vi "DB UI - Master Data Layout.vi"() -> ()   [LabVIEW 2013]
uses:
  Controls/Output Set Cluster.ctl
  Controls/Combo Box.ctl
  <vilib>/Utility/miscctls.llb/LVRowAndColumnUnsignedTypeDef.ctl
  <vilib>/Utility/miscctls.llb/LVRowAndColumnTypeDef.ctl
  <vilib>/Utility/miscctls.llb/LVPointTypeDef.ctl
  Controls/DB - Master Data Layout Enum.ctl
  Controls/DB - [MasterData].[OutputSet] ColNames.ctl
  Controls/Global SRTRS.vi
  <vilib>/addons/database/Connection.llb/DB Tools Open Connec (String).vi
  <vilib>/addons/database/Connection.llb/Conn Execute.vi
  <vilib>/addons/database/Recordset.llb/Rec Destroy - Connection.vi
  <vilib>/addons/database/Recordset.llb/Rec Fetch Recordset Data (R).vi
  <vilib>/addons/database/_DB Variant To Data/Database Variant To Data.xnode
  <vilib>/addons/database/NI_Database_API.lvlib
  Controls/Message Code - Enum.ctl
panel:
  in  "Tab Control":enum32{"Debug"}(tab)
  out "MHandler":errorcluster
  in  "Stop Button":bool
  out "Statemachine":errorcluster
  in  "# of Columns":i32=8
  out "Primary Keys":string[](array[string])=["OrderNo"]
  out "Foreign Keys":string[](array[string])=["OrderNo"]
  out "Record Count":i32
  in  "Next Button":bool
  in  "Previous Button":bool
  in  "Current Record":i32
  out "1st Primary KEY":string
  in  "Last Button":bool
  in  "First Button":bool
  out "datetime string":string
  out "Output Set Changed":bool
  in  "Include Inactive":bool=TRUE
  out "Extra Event From \"Select Foreign Key\" (NA)":bool
  out "IDENTITY COLUMN":string
  out "Close":errorcluster
  out "New Record in UI not in DB (NA)":bool
  out "Property Node":errorcluster
  out "DB":errorcluster
  in  "SRTRS.MasterData.OutputSet":string="SRTRS.MasterData.OutputSet"
  in  "[PlantId]":string="4070"
  in  "SRTRS.MasterData.OutputLayout":string="SRTRS.MasterData.OutputLayout"
  in  "SRTRS.Config.OutputType":string="SRTRS.Config.OutputType"
  out "Col Hdrs[] DB Data Type":string[](array[string])
  in  "Search User ID":T1
  in  "# of Rows":u32=5
  out "Col Hdrs[] DB Precision":string[](array[string])
  out "All Mandatory Fields Filled":bool
  in  "------------------------------------        Layout Details EVENTS     ------------------------------------":string caption="------------------------------------        Setup Tab     ------------------------------------"
  in  "------------------------------------------        Unused EVENTS     ----------------------------------------":string caption="------------------------------------        Setup Tab     ------------------------------------"
  out "Connection Information":T2={"Connection "="SQL Server 32bit HPEnvy", "Username"="admin", "Password"="admin123"}
  out "[Column Name] Changed":string
  out "File":errorcluster
  out "Editing Layout Details in New Record":bool
  in  "------------------------------------        Header EVENTS     ------------------------------------   2":string caption="------------------------------------        Setup Tab     ------------------------------------"
  in  "------------------------------------        MCListBox EVENTS     ------------------------------------   3":string caption="------------------------------------        Setup Tab     ------------------------------------"
  out "Precision":i32
  out "SQL":string[](array[string])
  in  "SRTRS.MasterData.Layout":string="SRTRS.MasterData.Layout"
  out "New Layout Id":string[](array[string])
  out "Source path":path caption="selected path"
  out "Target path":path
  out "File Copy Error":errorcluster
  out "MCListBox":u32
  out "NewVal":i32
  out "Layout Details":u32
  in  "Add (Not Save) Enabled depends on \nFilled Mandatory Fields":bool=TRUE
  out "Empty ColHdrs[]":string[](array[string])
  in  "UPDATE ALL LayoutId":bool=TRUE
  in  "CellBG New Cells":u32(colorbox)=16777225
  in  "CellBG Unused Cells":u32(colorbox)=16777238
  in  "CellBG ColHdrs":u32(colorbox)=11776947
  in  "New Layout ID":bool
  in  "Output Set Header":T3 caption="Header"
  in  "Layout Browse":bool caption="Material Browse"
  in  "Item Number":i32=1 min=0 step=1
  in  "Layout Details Cluster":T4 caption="Layout Details"
  in  "Delete":bool caption="Setup Save"
  in  "Add":bool caption="Setup Save"
  in  "Save":bool caption="Setup Save"
  in  "New":bool caption="Setup Save"
  in  "MCListbox Layout":i32(listbox)=3 caption="MCListBox Layout"
  # "No."
  # "/"
  # "Record"
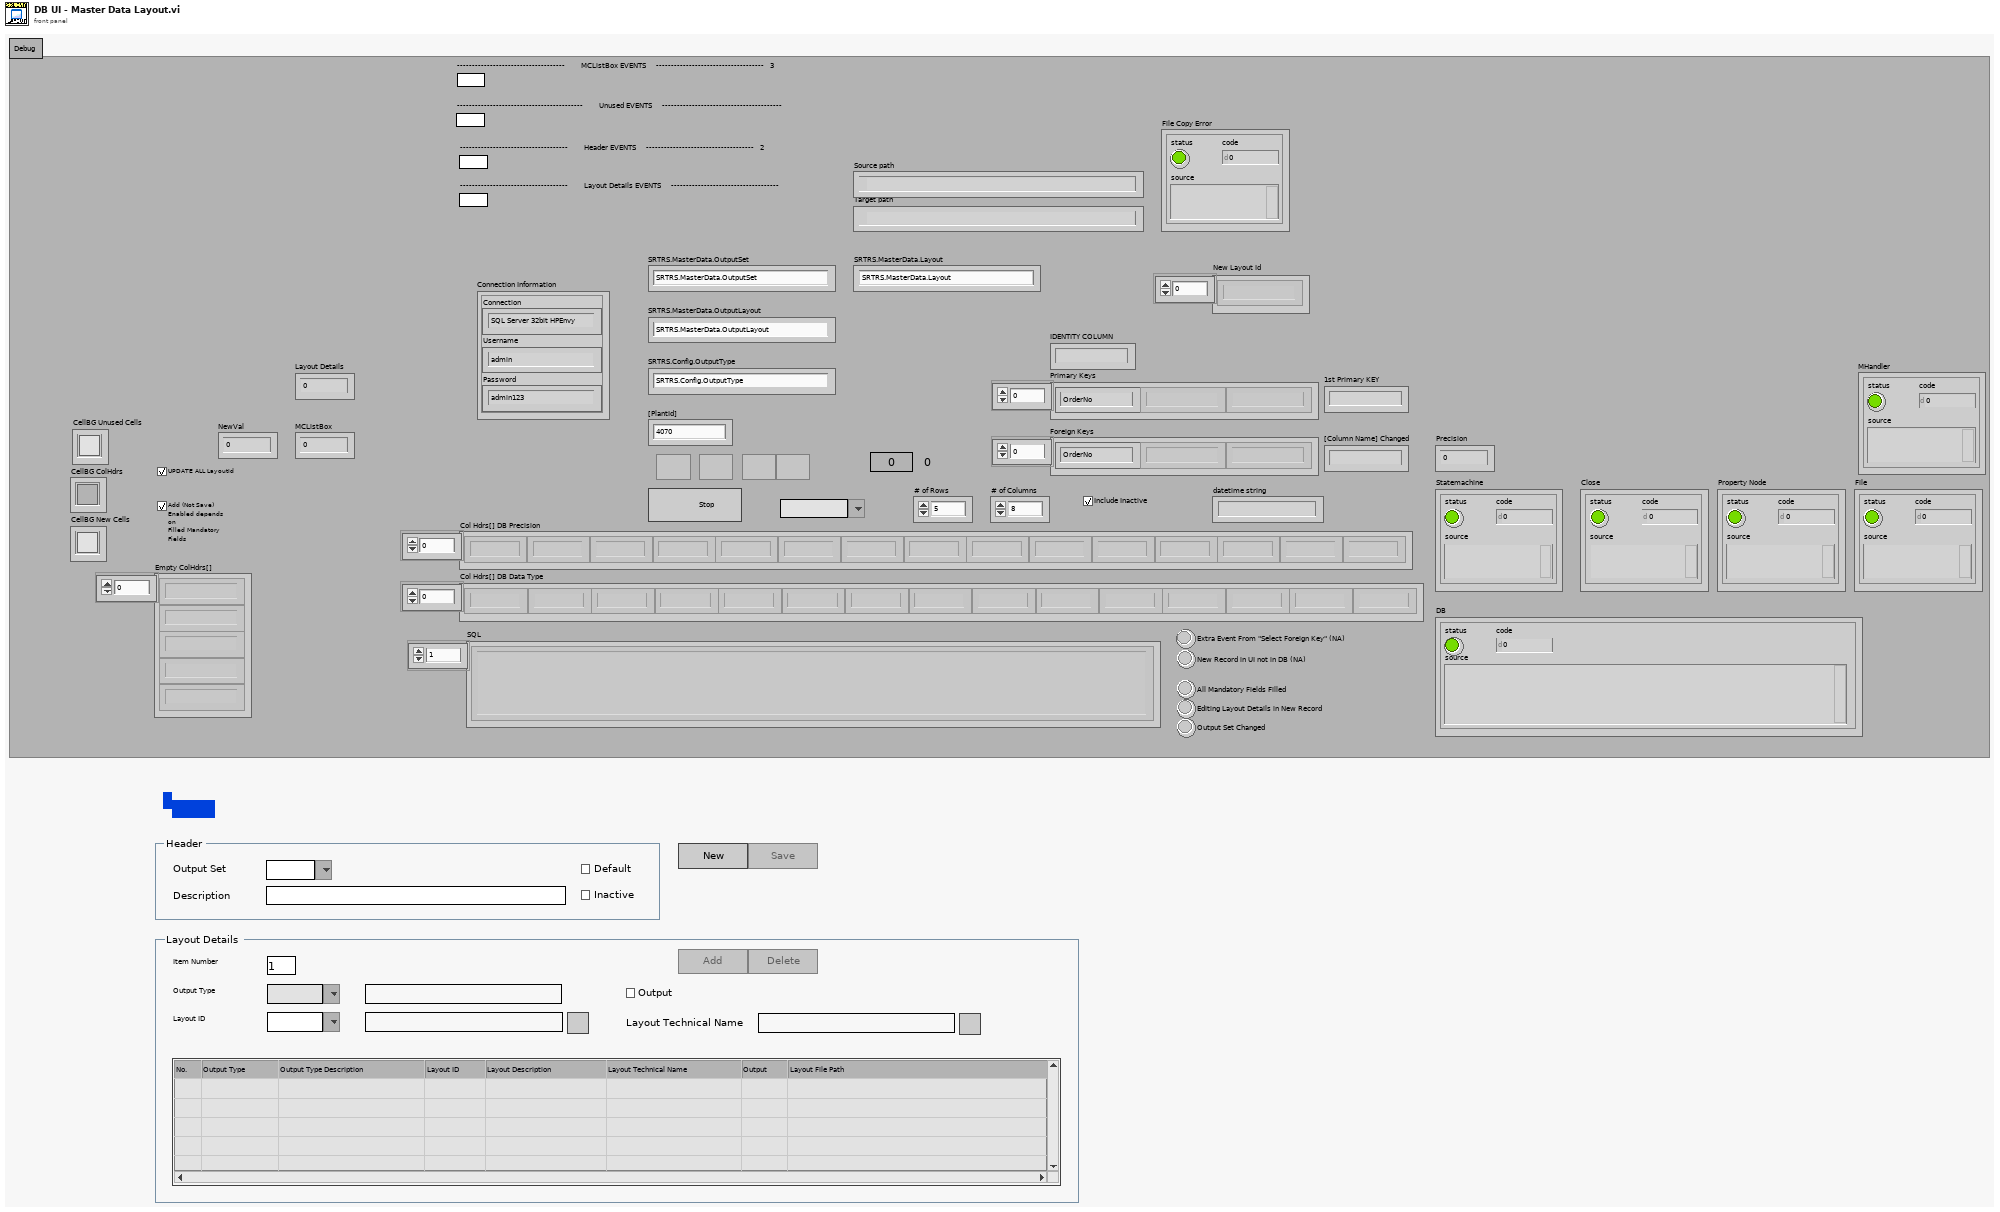
[diagram p1: front panel]
types:
  T1 = typedef "Combo Box.ctl" = string
  T2 = cluster{"Connection ":string, "Username":string, "Password":string}
  T3 = typedef "Output Set Cluster.ctl" = cluster{"Output Set":T1, "Description":string, "Default":bool, "Inactive":bool}
  T4 = cluster{"Output Type":T1, "Output":bool, "Inactive":bool, "Layout Description":string, "Layout ID":T1, "Layout Technical Name":string, "Output Type Description":string, "Layout File Path":string}
  T5 = enum8{"Enabled", "Disabled", "Disabled and Grayed Out"}
  T6 = typedef "LVPointTypeDef.ctl" = cluster{"Horizontal":i16, "Vertical":i16}
  T7 = typedef "LVRowAndColumnUnsignedTypeDef.ctl" = cluster{"Row":u32, "Column":u32}
  T8 = typedef "DB - Master Data Layout Enum.ctl" = enum16{"b.[ItemNo]", "a.[OutputSetId]", "a.[Description]", "a.[Default]", "a.[Inactive]", "b.[OutputTypeId]", "c.[ShortDescription]", "b.[Output]", "b.[Inactive]", "b.[LayoutId]", "b.[Description]", "b.[LayoutFileName]", "b.[LayoutFilePath]"}
  T9 = typedef "LVRowAndColumnTypeDef.ctl" = cluster{"Row":i32, "Column":i32}
  T10 = typedef "DB - Logon Info.ctl" = cluster{"PlantID":string, "SystemID":string, "UserID":string, "DomainID":string, "LanguageID":string, "StationID":string}
  T11 = typedef "Connection Information Cluster.ctl" = cluster{"Connection ":string, "Username":string, "Password":string}
  T12 = typedef "NI_Database_API.lvlib/Conn ObjectReference.ctl" = refnum<k1>
  T13 = typedef "Message Code - Enum.ctl" = enum16{"<APP><I 100>", "<APP><E 101>", "<APP><I 110>", "<APP><W 111>", "<APP><I 112>", "<APP><W 113>", "<APP><I 114>", "<APP><I 115>", "<APP><I 116>", "<APP><W 117>", "<APP><I 120>", "<APP><W 121>", "<APP><E 122>", "<APP><W 130>", "<APP><W 131>", "<APP><W 132>", "<APP><W 133>", "<APP><W 134>", "<DB><I 150>", "<DB><I 151>", "<DB><W 152>", "<APP><I 200>", "<APP><I 201>", "<APP><W 202>", "<APP><E 203>", "<DB><I 300>", "<DB><I 301>", "<DB><W 302>", "<DB><I 305>", "<DB><I 306>", "<DB><W 307>", "<DB><W 310>", "<cRIO><I 400>", "<cRIO><W 401>", "<cRIO><I 402>", "<cRIO><W 403>", "<ET><I 500>", "<ET><W 501>", "<ET><I 600>", "<ET><W 601>", "<ET><E 602>", "<ET><I 610>", "<ET><W 611>", "<ET><E 612>"}
  T14 = typedef "DB - [MasterData].[OutputSet] ColNames.ctl" = enum16{"[PlantId]", "[OutputSetId]", "[Description]", "[Default]", "[CreatedBy]", "[CreatedOn]", "[LastSavedBy]", "[LastSavedOn]", "[Inactive]"}
  T15 = typedef "DB - DB.Schema.Table.ctl" = cluster{"DB":string, "Schema":string, "Table":string}
  T16 = typedef "NI_Database_API.lvlib/Rec ObjectReference.ctl" = refnum<k1>
  T17 = cluster{"Output Set":T1, "Description":string, "Default":bool, "Inactive":bool}
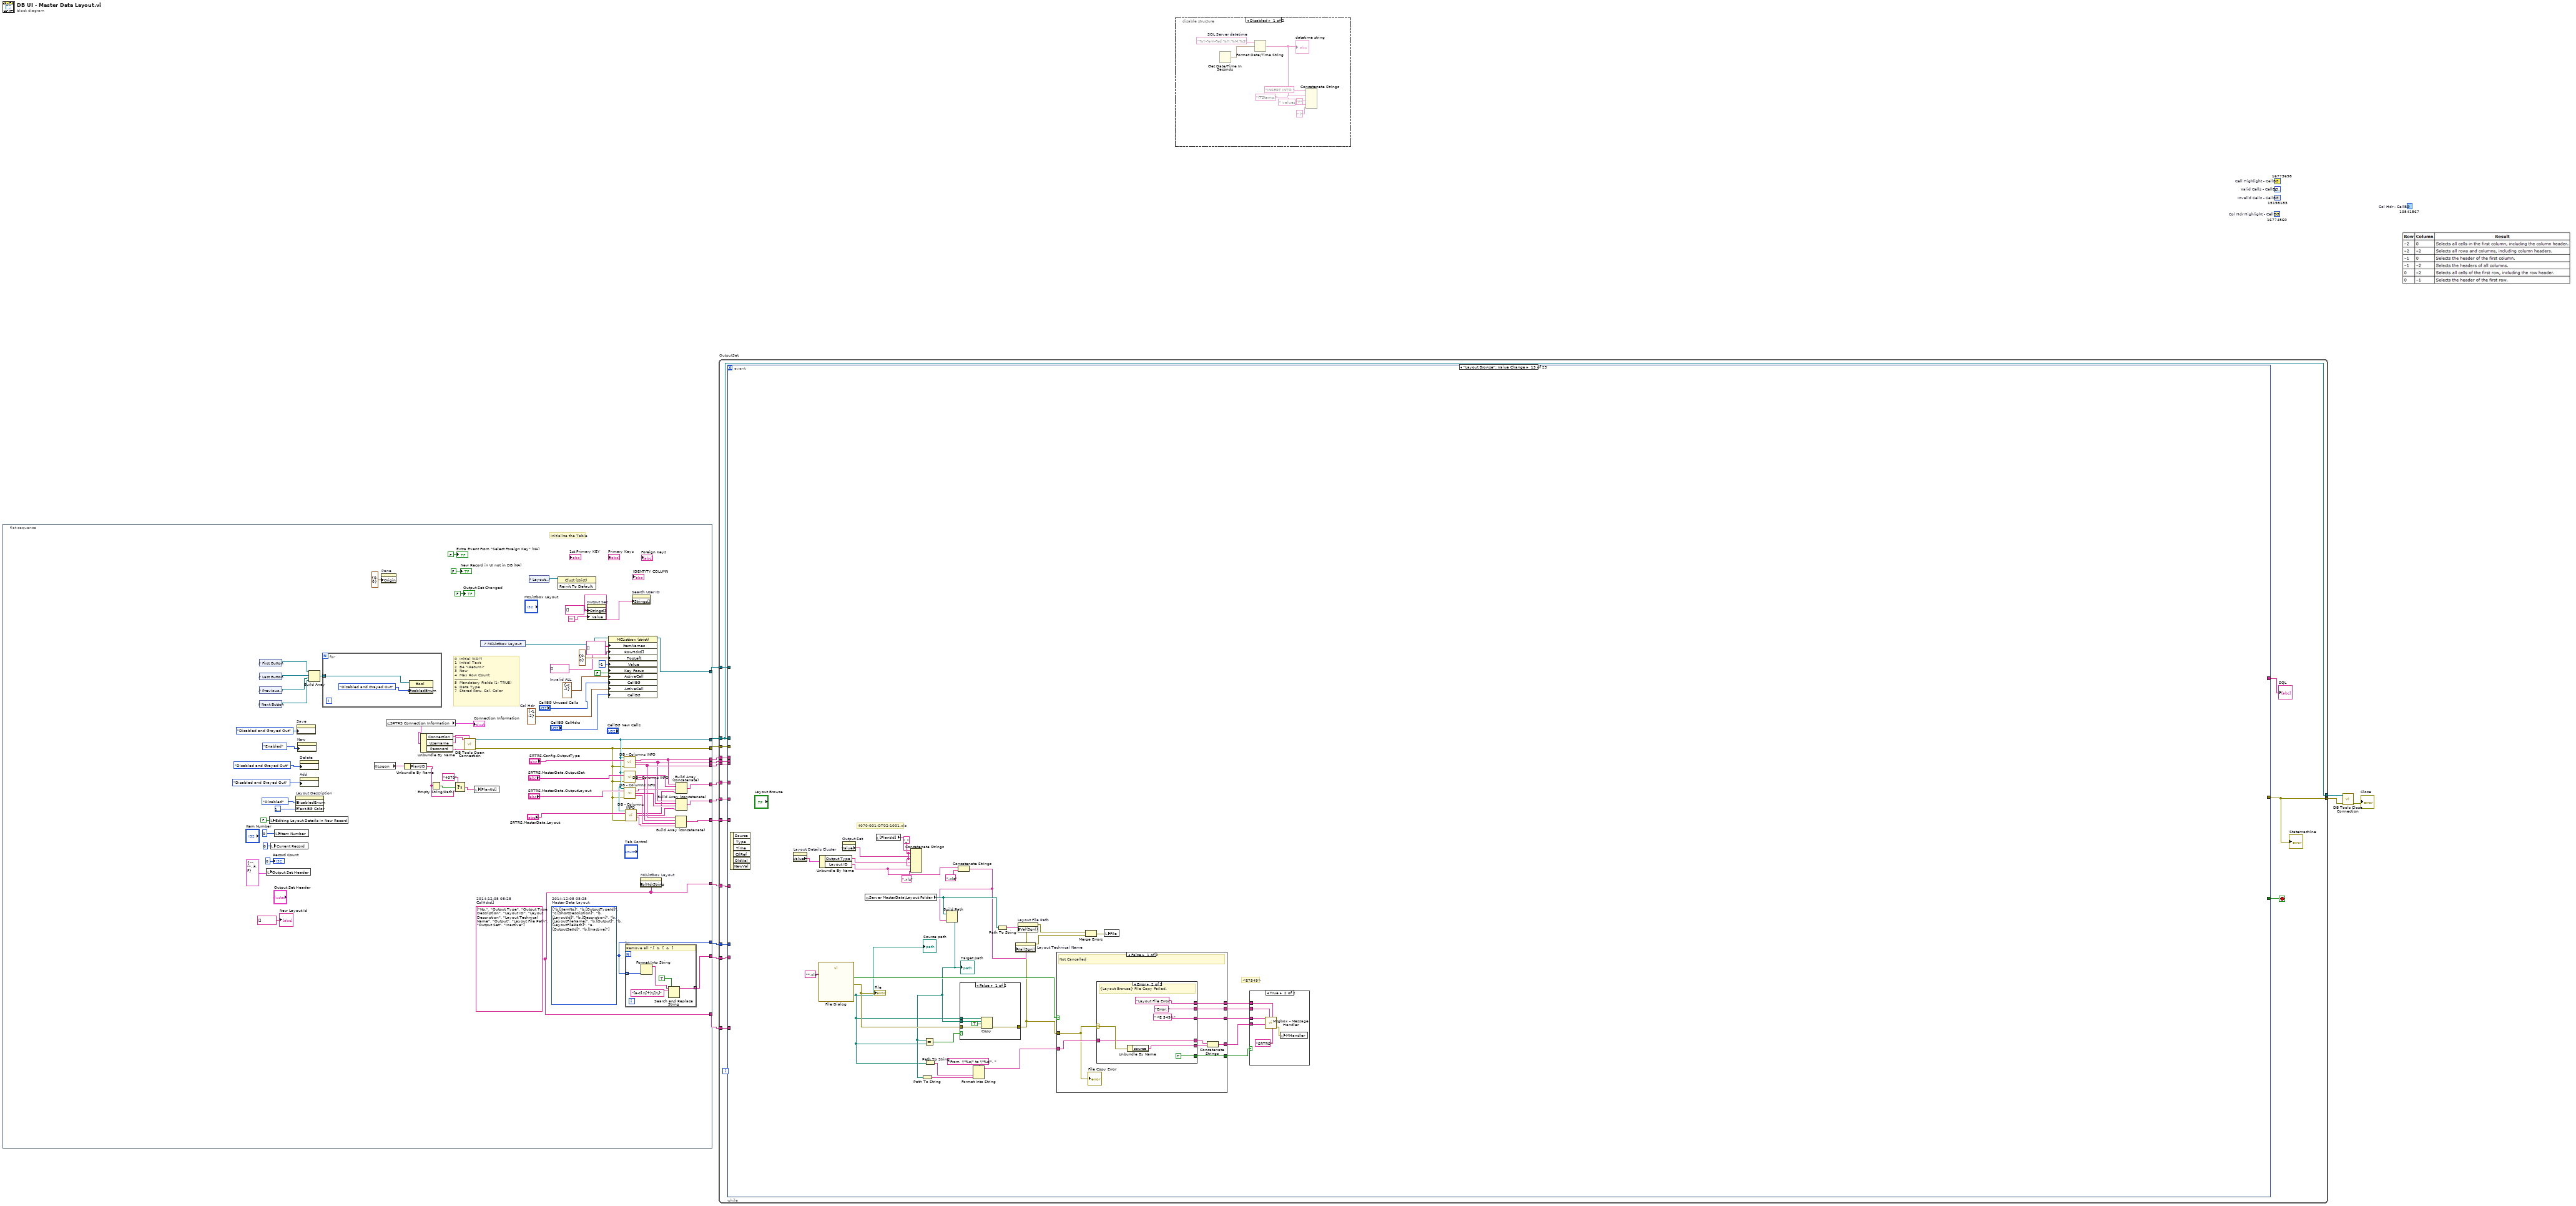
[diagram p0: block diagram]
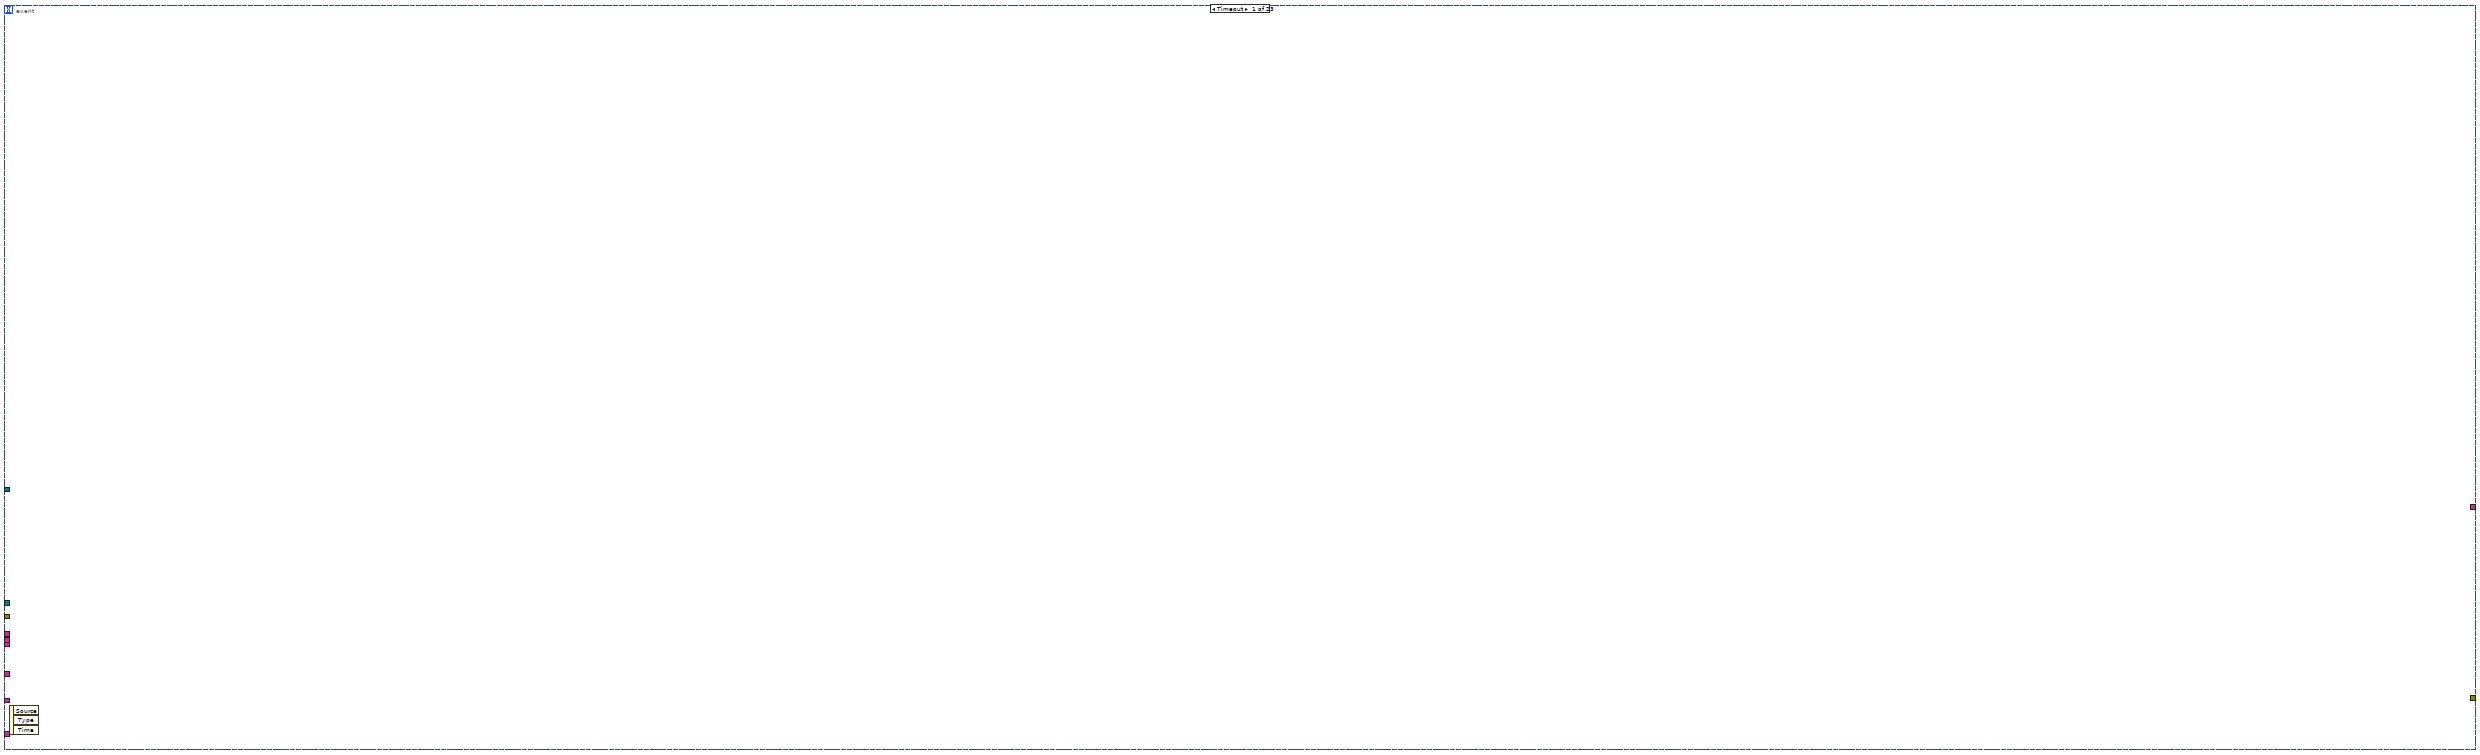
[diagram p3: hidden frame]
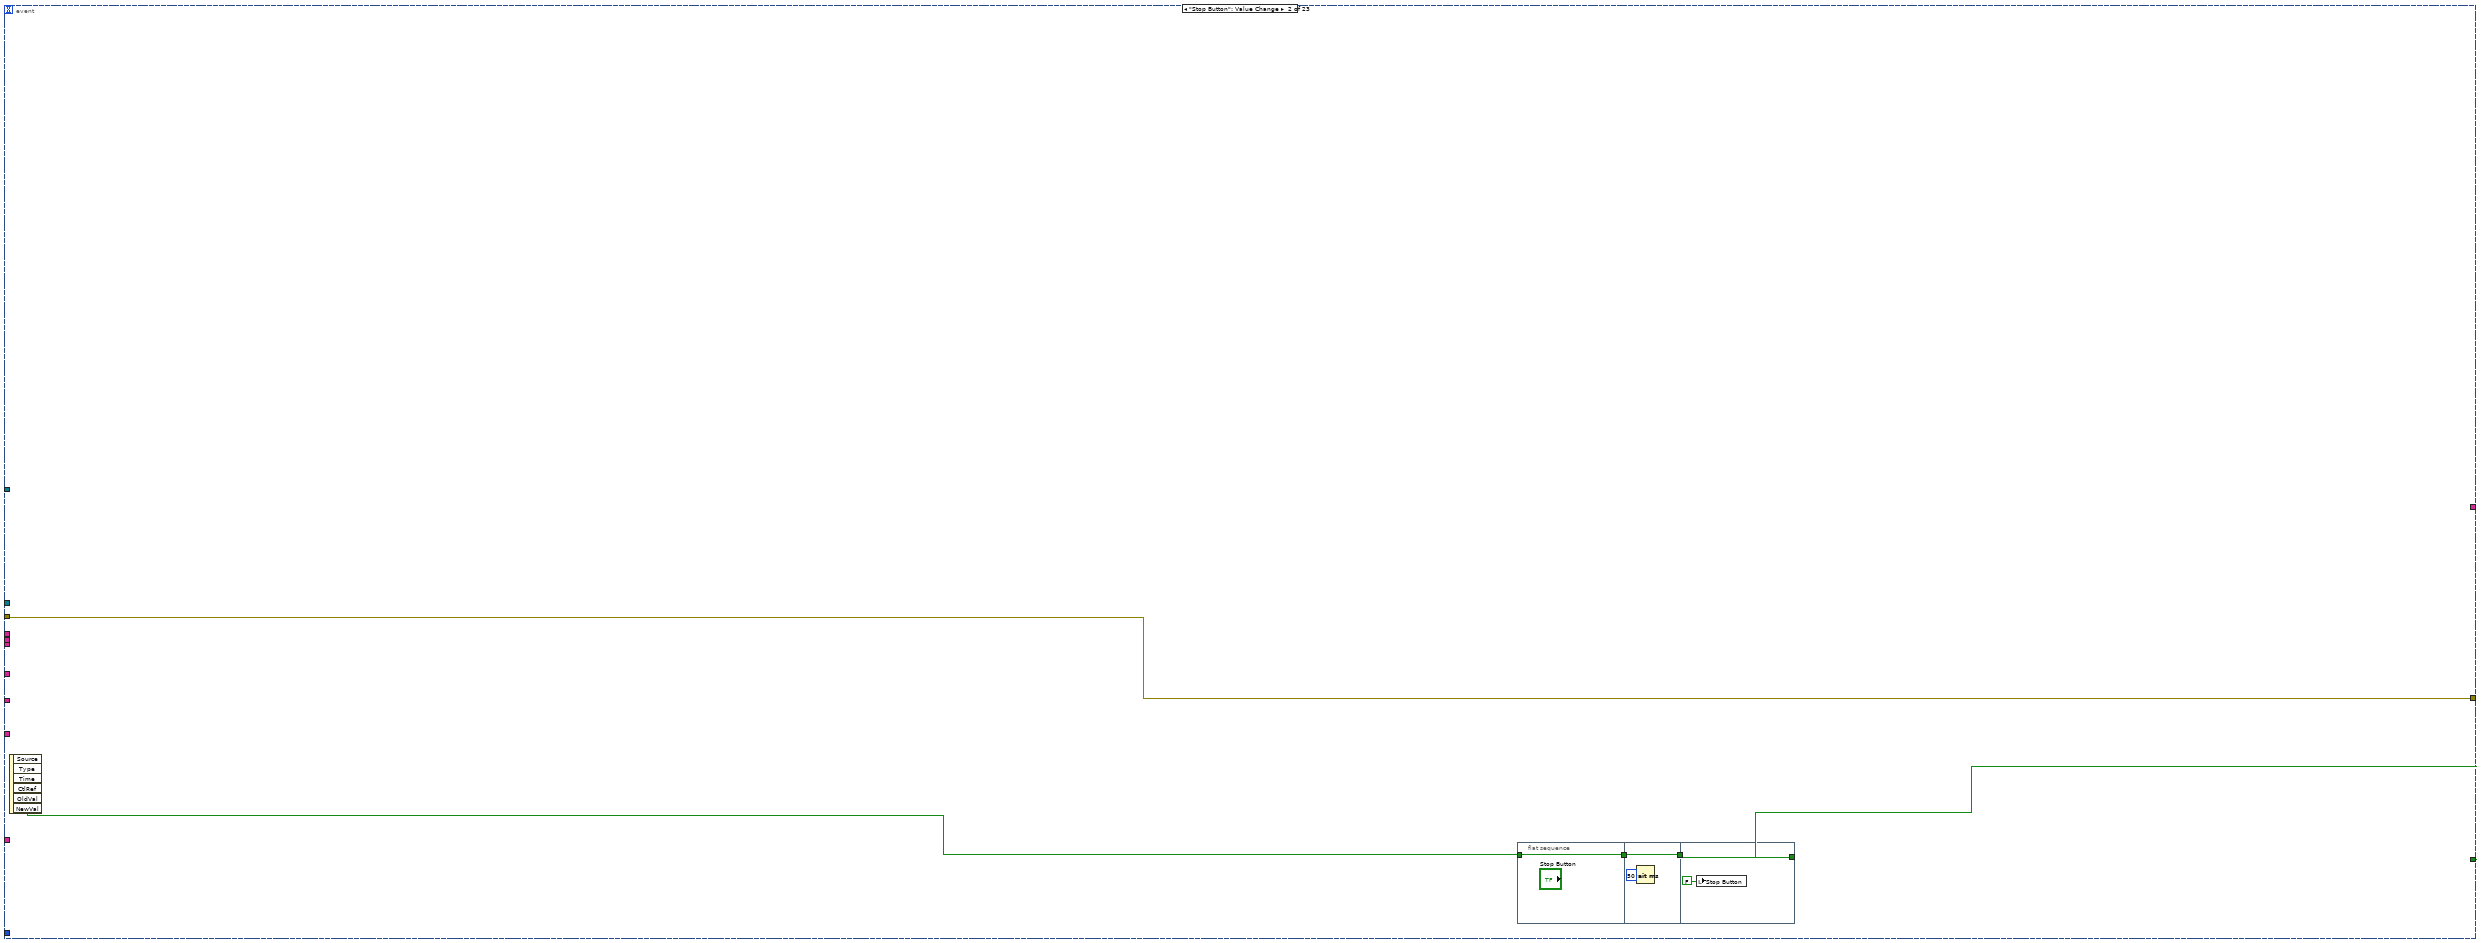
[diagram p4: hidden frame]
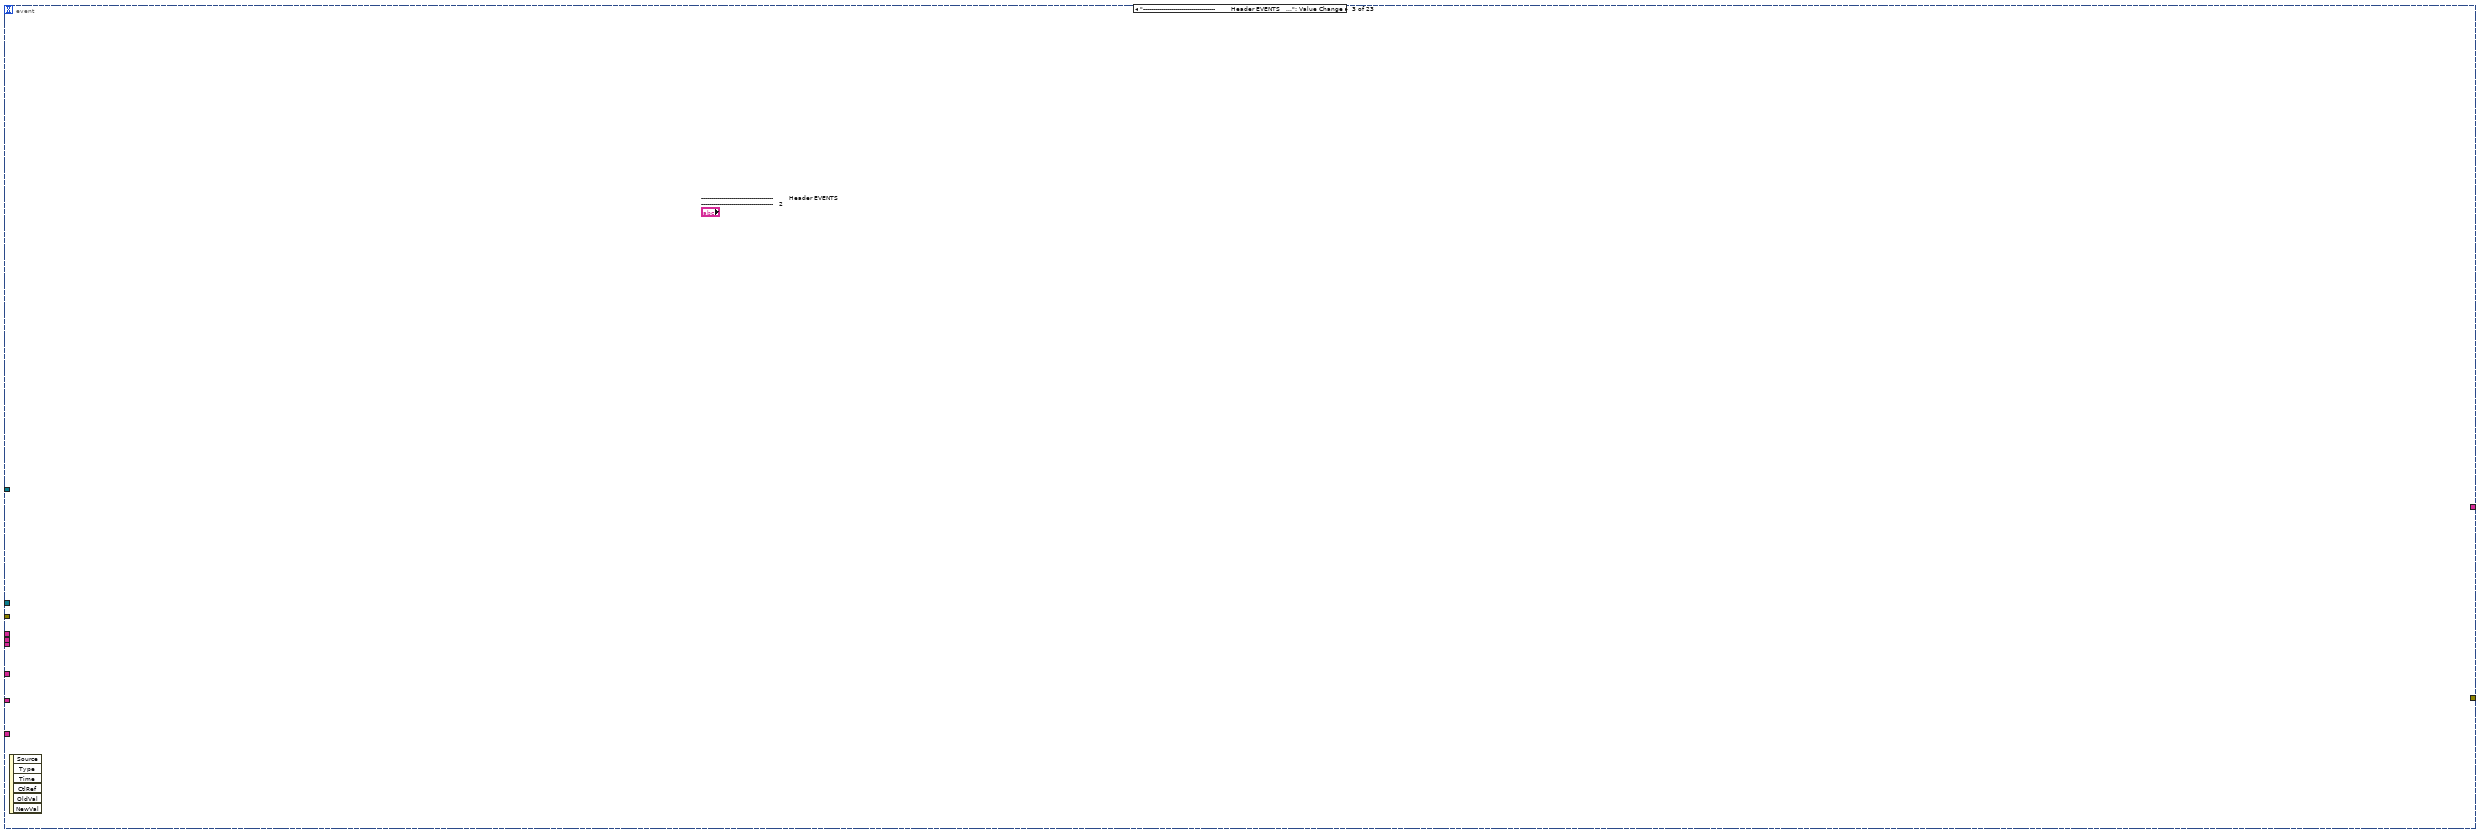
[diagram p5: hidden frame]
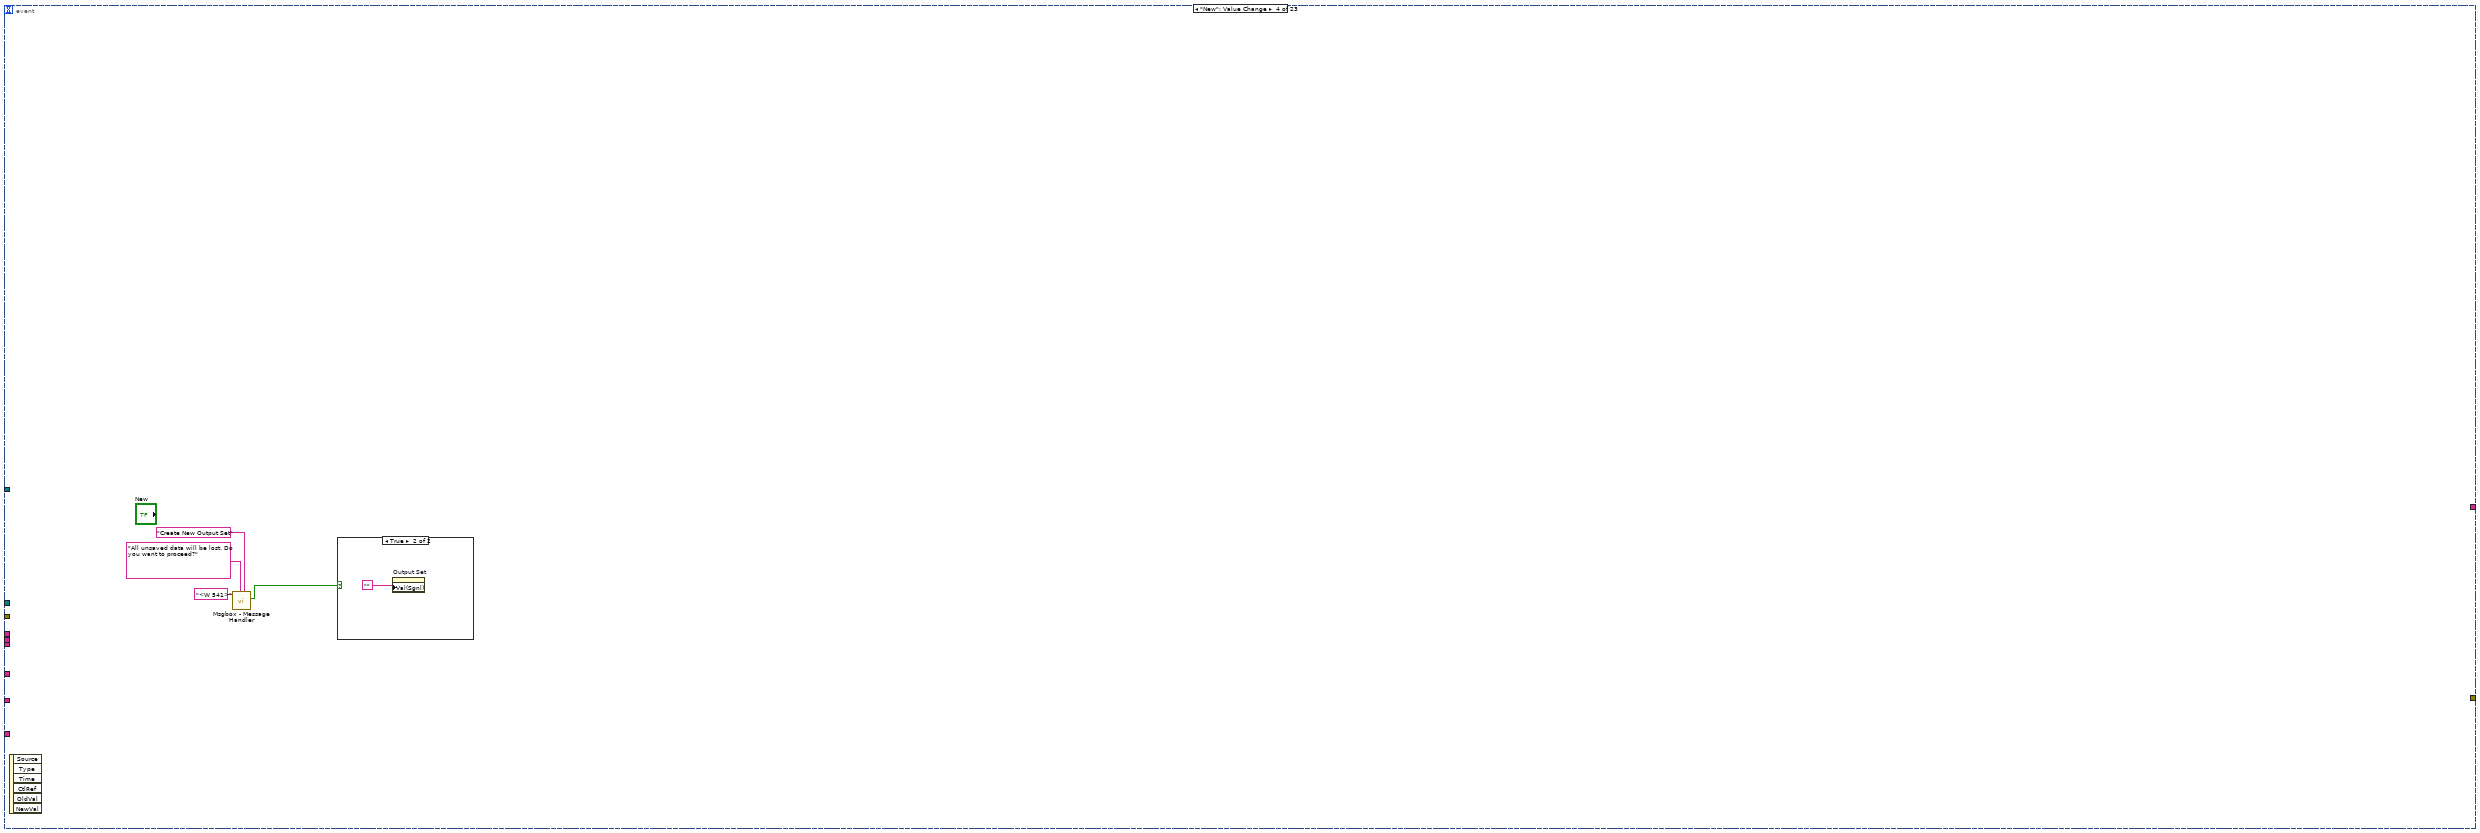
[diagram p6: hidden frame]
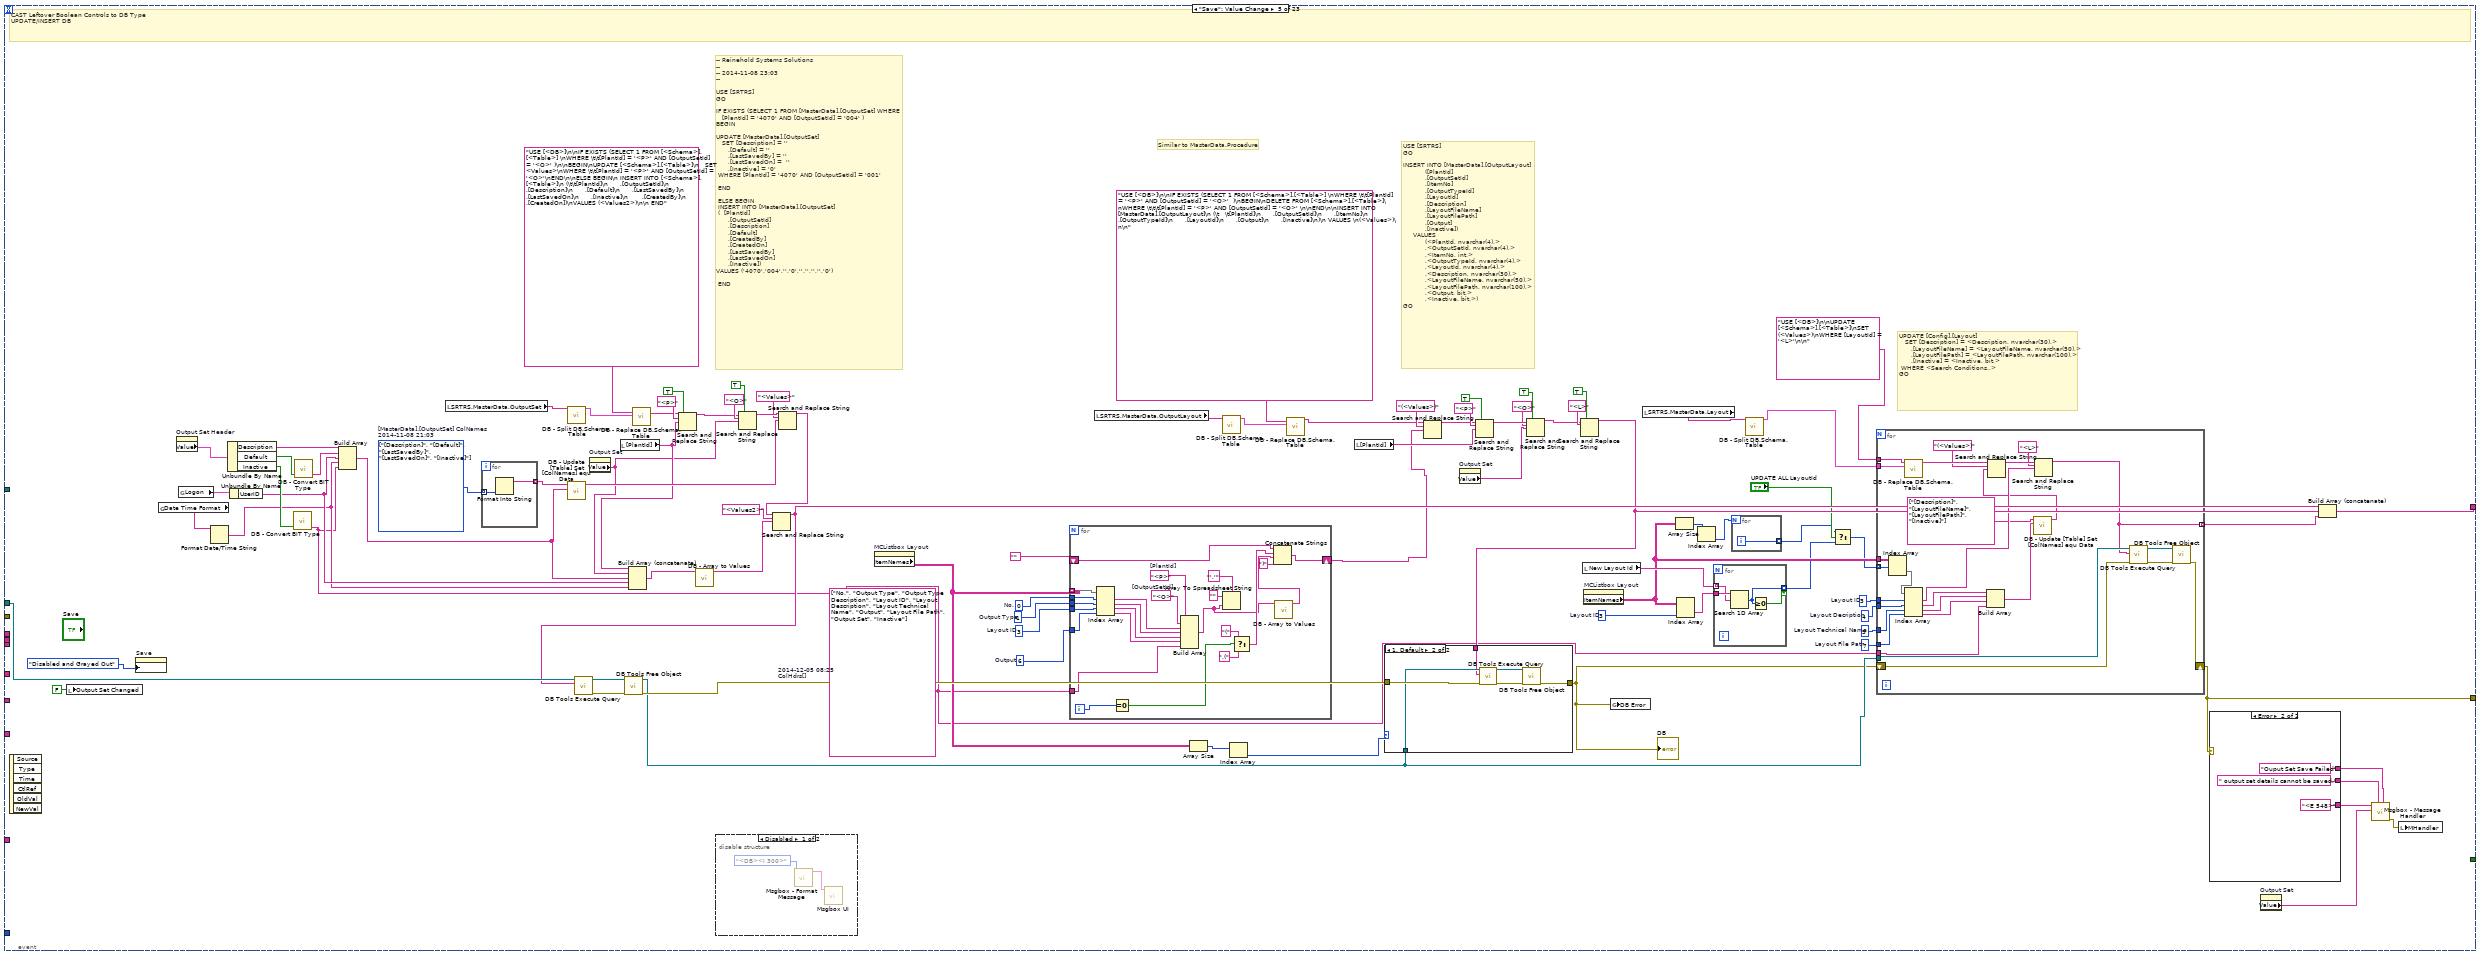
[diagram p8: hidden frame]
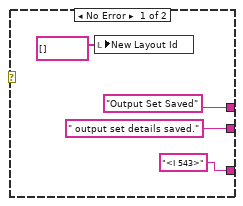
[diagram p9: hidden frame]
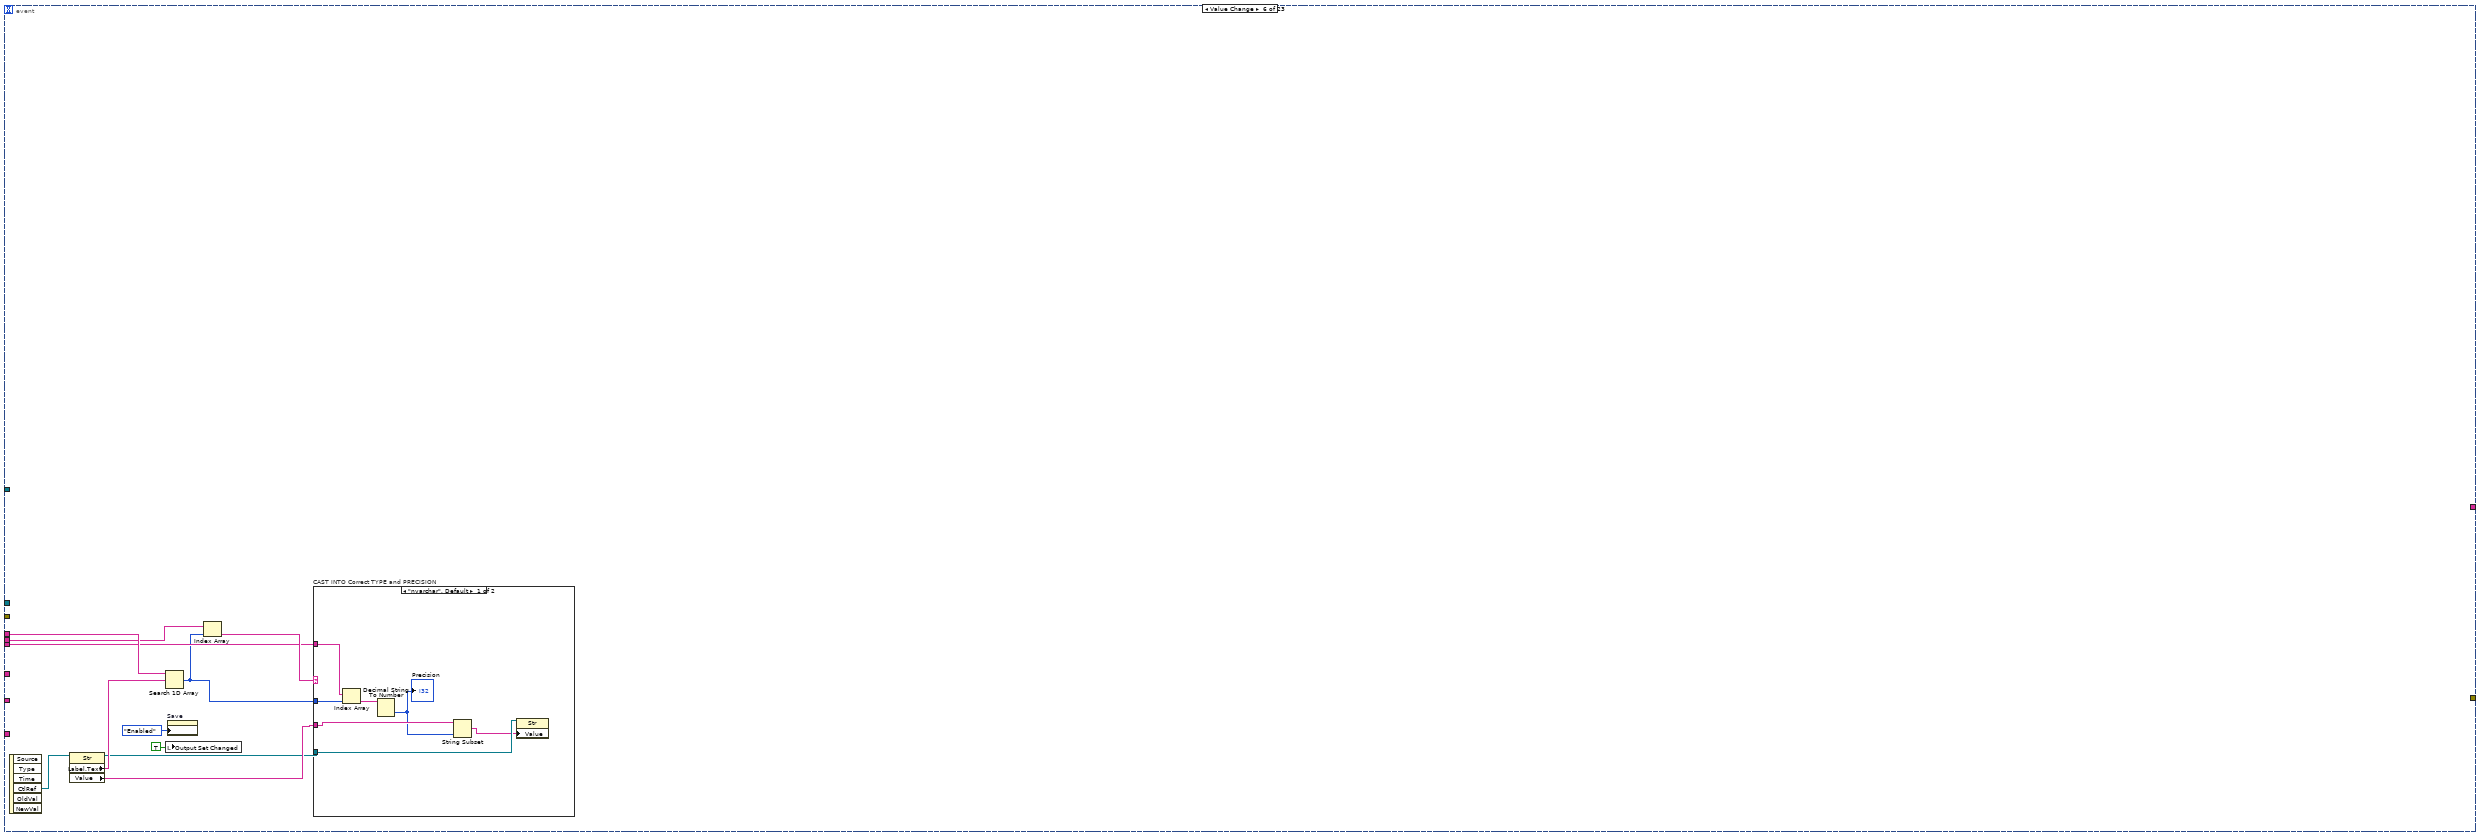
[diagram p12: hidden frame]
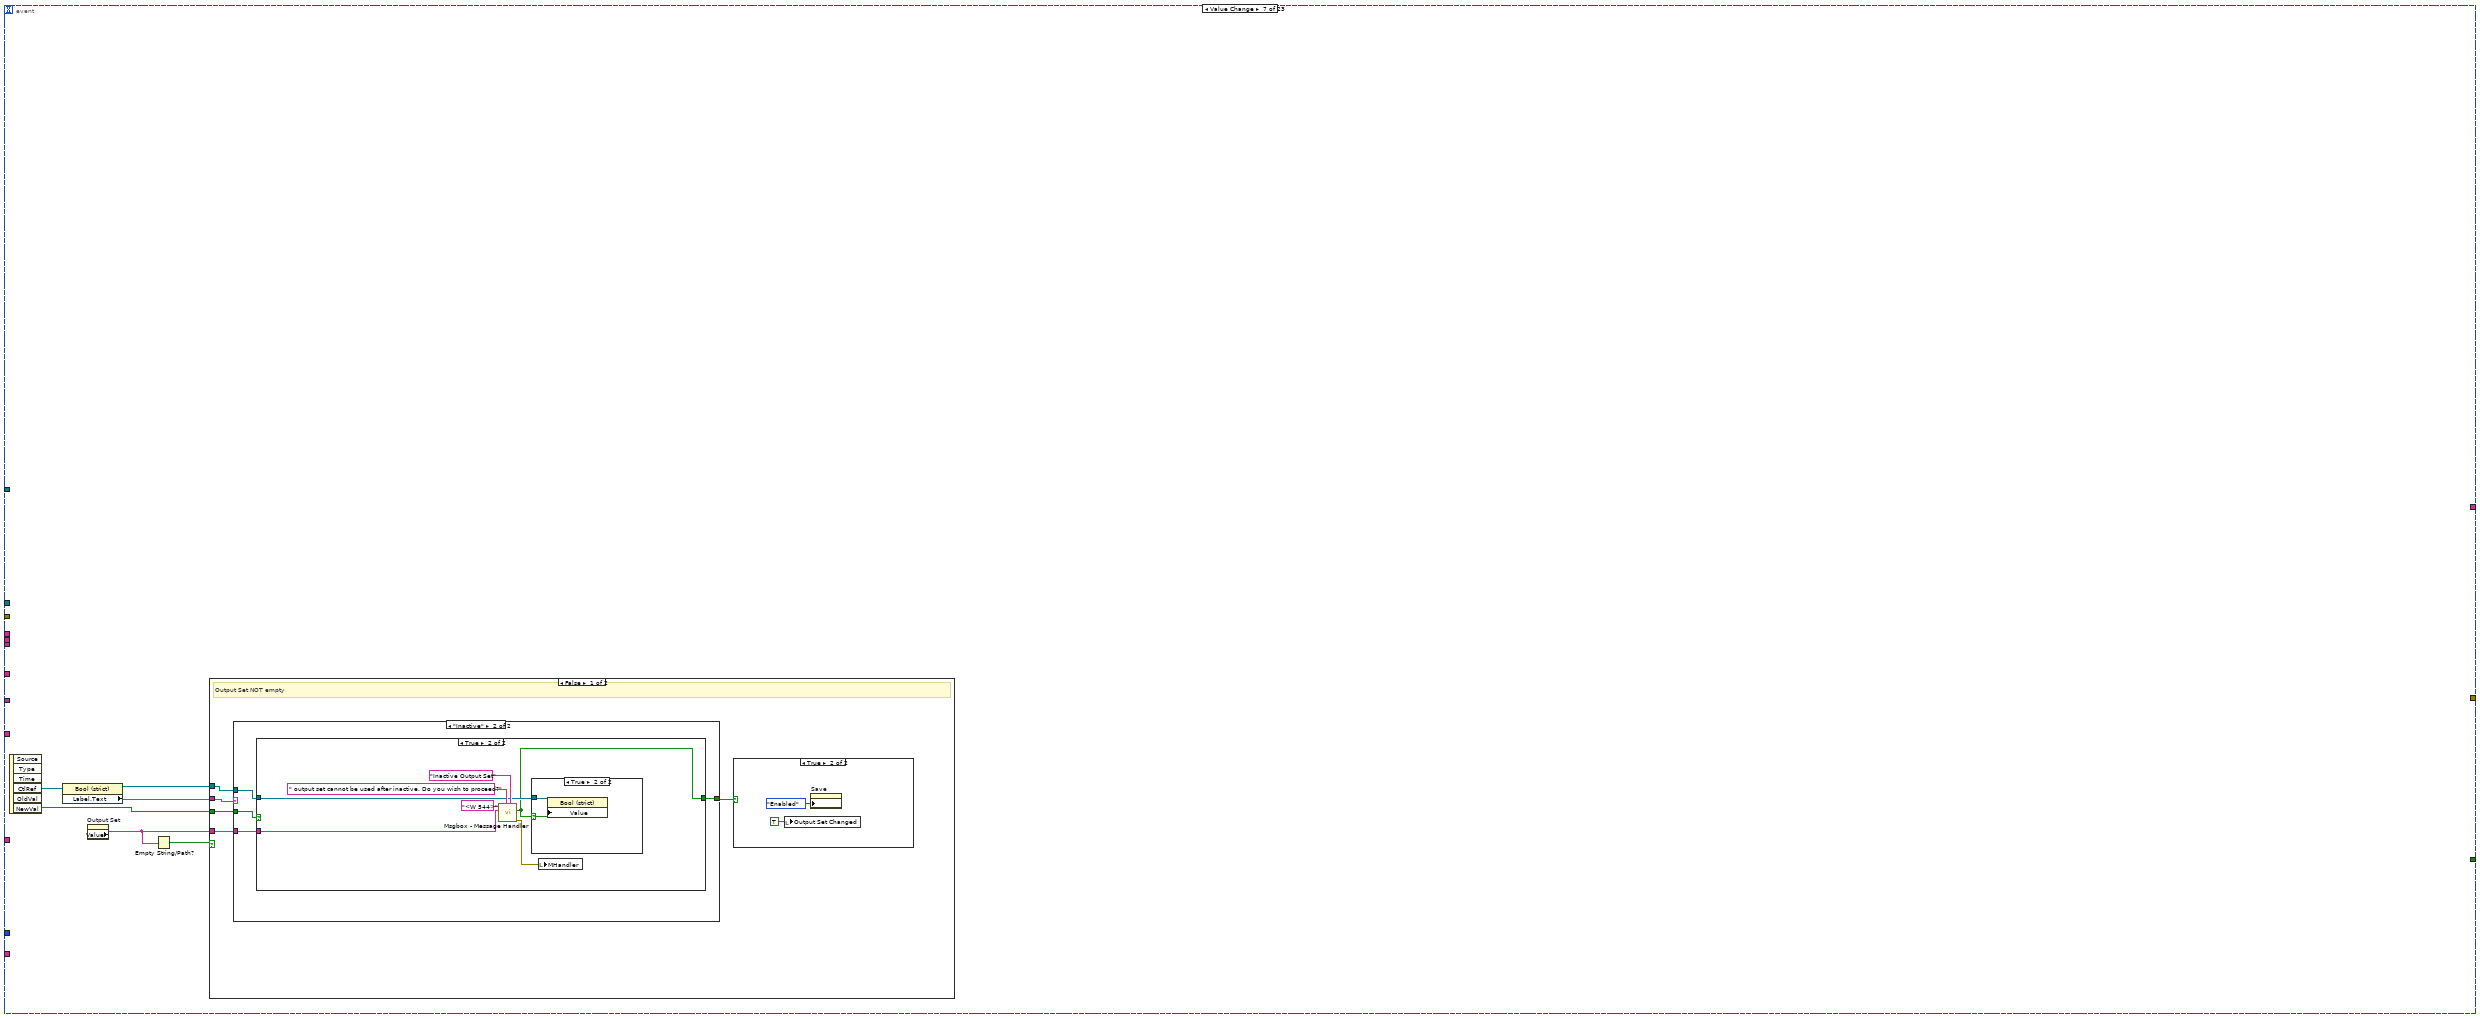
[diagram p14: hidden frame]
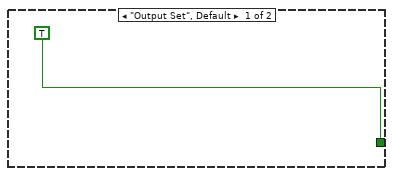
[diagram p16: hidden frame]
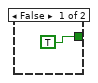
[diagram p17: hidden frame]
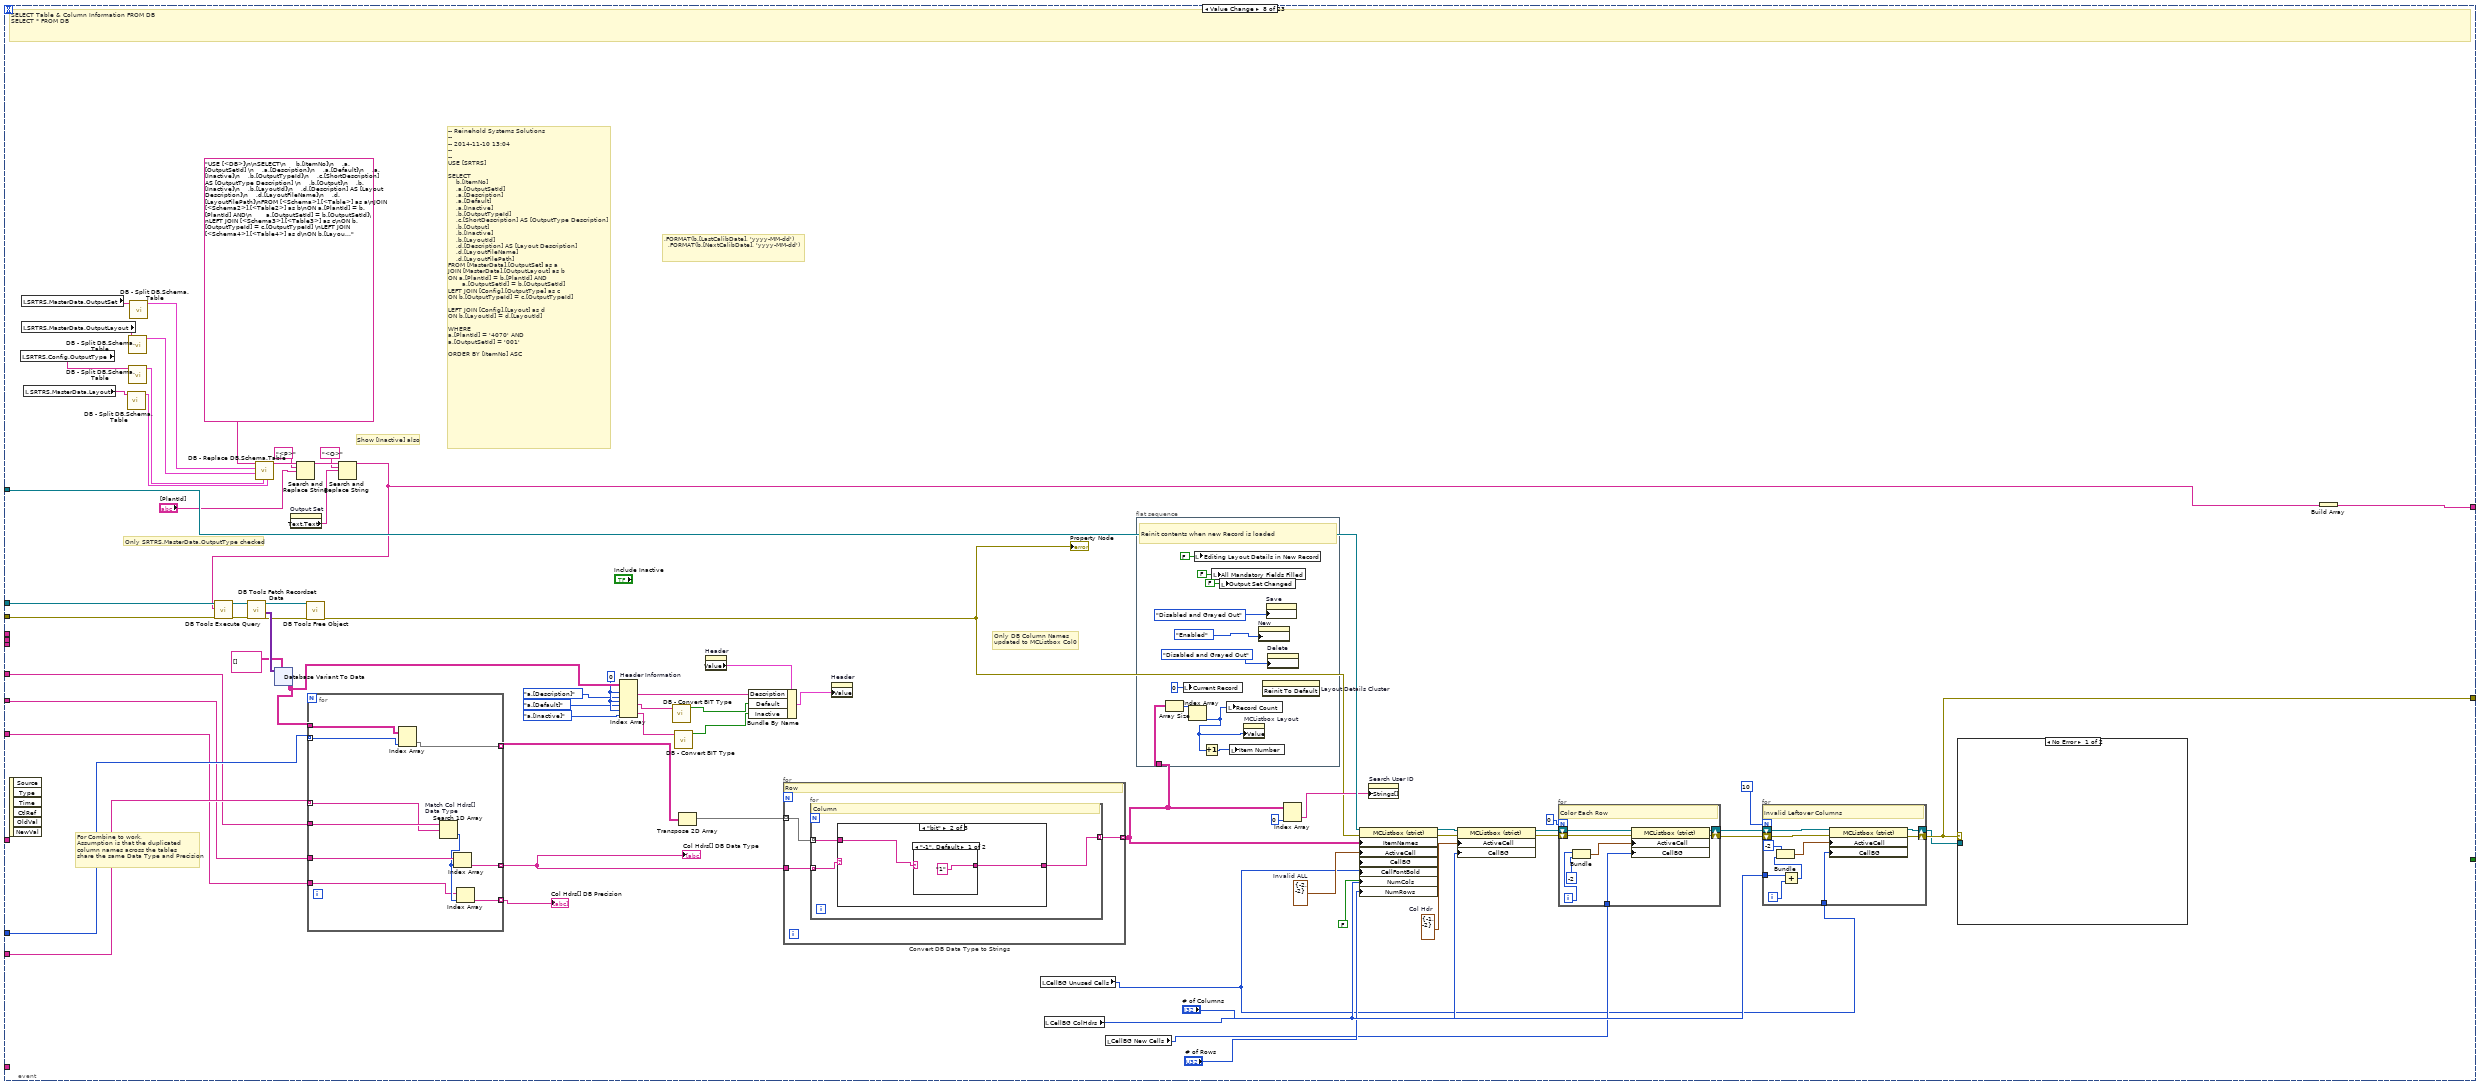
[diagram p20: hidden frame]
diagram:
  (unwired) u32 10541567  # Col Hdr - CellBG
  (unwired) u32 16777226  # Valid Cells - CellBG
  (unwired) u32 15198183  # Invalid Cells - CellBG
  (unwired) u32 16774560  # Col Hdr Highlight - CellBG
  (unwired) u32 16773698  # Cell Highlight - CellBG
  n1 = flat-sequence {
    tunnel: [w26] -> w16
    tunnel: [w65] -> w13
    tunnel: [w25] -> w12
    tunnel: [w60] -> w10
    tunnel: [w52] -> w9
    tunnel: [w59] -> w8
    tunnel: [w52] -> w7
    tunnel: [w41] -> w6
    tunnel: [w40] -> w5
    tunnel: [w39] -> w4
    tunnel: [w35] -> w3
    tunnel: [w34] -> w2
    tunnel: [w33] -> w1
    frame #0 {
      w59 = T8[] [enum."b.[ItemNo]", enum."b.[OutputTypeId]", enum."c.[ShortDescription]", enum."b.[LayoutId]", enum."b.[Description]", enum."b.[LayoutFileName]", enum."b.[Output]", enum."b.[LayoutFilePath]", enum."a.[OutputSetId]", enum."b.[Inactive]"] items=["b.[ItemNo]", "a.[OutputSetId]", "a.[Description]", "a.[Default]", "a.[Inactive]", "b.[OutputTypeId]", "c.[ShortDescription]", "b.[Output]", "b.[Inactive]", "b.[LayoutId]", "b.[Description]", "b.[LayoutFileName]", "b.[LayoutFilePath]"]  # 2014-12-05 08:25 Master Data Layout
      w62 = string[] [] ("Strings []")
      w52 = string[] ["No.", "Output Type", "Output Type Description", "Layout ID", "Layout Description", "Layout Technical Name", "Output", "Layout File Path", "Output Set", "Inactive"]  # 2014-12-05 08:25 ColHdrs[]
      w66 = T9 {"Row"=-1, "Column"=-2}  # Col Hdr
      w67 = T9 {"Row"=-2, "Column"=-2}  # Invalid ALL
      # "15"
      # "10"
      # "5"
      # "Initialize the Table"
      # "0  Initial (KD?)\n1  Initial Text\n2  B4 <Return>\n3  Now\n4  Max Row Count\n-------------------\n5  Mandatory Fields (1- TRUE)\n6  Data Type\n7  Stored Row, Col, Color"
      n2 = control-ref of="First Button"() -> (w78:refnum<vi>)
      n3 = control-ref of="Last Button"() -> (w77:refnum<vi>)
      n4 = control-ref of="Previous Button"() -> (w76:refnum<vi>)
      n5 = control-ref of="Next Button"() -> (w75:refnum<vi>)
      n6 = local write "Output Set Header"(T3 {"Output Set"="", "Description"="", "Default"=FALSE, "Inactive"=FALSE} ("Header")) -> ()
      n7 = local write "Editing Layout Details in New Record"(FALSE ("Editing Layout Details in New Record")) -> ()
      n8 = local write "Current Record"(0 ("Current Record")) -> ()
      n9 = local write "Item Number"(0 ("Current Record")) -> ()
      n10 = property on="Layout Description" class="Str"("DisabledEnum"=T5."Disabled" ("Disabled"), "Text.BG Color"=u32 16777216) -> ()  [unwired: 2 in, 2 out]
      n11 = property on="Save" class="Bool"("DisabledEnum"=T5."Disabled and Grayed Out" ("Disabled")) -> ()  [unwired: 2 in, 2 out]
      n12 = property on="New" class="Bool"("DisabledEnum"=T5."Enabled" ("Disabled")) -> ()  [unwired: 2 in, 2 out]
      n13 = property on="Delete" class="Bool"("DisabledEnum"=T5."Disabled and Grayed Out" ("Disabled")) -> ()  [unwired: 2 in, 2 out]
      n14 = property on="Add" class="Bool"("DisabledEnum"=T5."Disabled and Grayed Out" ("Disabled")) -> ()  [unwired: 2 in, 2 out]
      n15 = Build Array(w78, w77, w76, w75) -> (w79:refnum<vi>[])
      n16 = for {
        tunnel: w79 -> [w91] mode=indexing
        n17 = property class="Bool"(reference=w91, "DisabledEnum"=T5."Disabled and Grayed Out" ("Disabled")) -> ()  [unwired: 1 in, 2 out]
      }
      n18 = global read "Global SRTRS.vi" "Logon"() -> (w32:T10)
      n19 = property on="Pane" class="Pane"("Origin"=T6 {"Horizontal"=0, "Vertical"=0}) -> ()  [unwired: 2 in, 2 out]
      n20 = global read "Global SRTRS.vi" "SRTRS Connection Information"() -> (w58:T11)
      "Connection Information" <- w58
      n21 = Unbundle By Name(w32) -> ("PlantID"=w28:string)
      n22 = Unbundle By Name(w58) -> ("Connection"=w84:string, "Username"=w83:string, "Password"=w82:string)
      n23 = Empty String/Path?(string/path=w28) -> (empty?=w31:bool)
      n24 = Select(t="4070", s=w31, f=w28) -> (s? t:f=w29:string)
      n25 = call-poly <vilib>:"DB Tools Open Connection.vi"("password"=w82, "userID"=w83, "connection information"=w84) -> ("error out"=w25:errorcluster, "connection reference"=w26:T12)  [unwired: 5 in]
      n26 = local write "[PlantId]"(w29) -> ()
      n27 = control-ref of="MCListbox Layout"() -> (w64:refnum<vi>)
      n28 = control-ref of="Layout Details Cluster"() -> (w63:refnum<vi>)
      n29 = invoke class="Clust (strict)" method="Reinit To Default"(reference=w63) -> ()  [unwired: 2 in, 3 out]
      n30 = property on="Output Set" class="CmbBox (strict)"("Strings[]"=w62, "Value"="") -> ()  [unwired: 2 in, 2 out]
      n31 = property on="Property Node" class="MCListbox (strict)"(reference=w64, "ItemNames"=string[][] [] ("Item Names"), "RowHdrs[]"=string[] [] ("Item Names"), "TopLeft"=T7 {"Row"=0, "Column"=0} ("Top Left Visible Cell"), "Value"=-1, "Key Focus"=FALSE, "ActiveCell"=w67, "CellBG"="CellBG Unused Cells", "ActiveCell"=w66, "CellBG"="CellBG ColHdrs") -> (reference out=w65:refnum<vi>)  [unwired: 1 in, 1 out]
      n32 = call "DB - Columns INFO.vi"("Refnum in"=w26, "DB.dbo.Table"="SRTRS.Config.OutputType", "error in (no error)"=w25) -> ("COLUMN_NAME"=w35:string[], "DATA_TYPE"=w33:string[], "PRECISION"=w34:string[])  [unwired: 4 in, 6 out]
      n33 = call "DB - Columns INFO.vi"("Refnum in"=w26, "DB.dbo.Table"="SRTRS.MasterData.OutputSet", "error in (no error)"=w25) -> ("COLUMN_NAME"=w42:string[], "DATA_TYPE"=w44:string[], "PRECISION"=w46:string[])  [unwired: 4 in, 6 out]
      n34 = call "DB - Columns INFO.vi"("Refnum in"=w26, "DB.dbo.Table"="SRTRS.MasterData.OutputLayout", "error in (no error)"=w25) -> ("COLUMN_NAME"=w43:string[], "DATA_TYPE"=w45:string[], "PRECISION"=w47:string[])  [unwired: 4 in, 6 out]
      n35 = call "DB - Columns INFO.vi"("Refnum in"=w26, "DB.dbo.Table"="SRTRS.MasterData.Layout", "error in (no error)"=w25) -> ("COLUMN_NAME"=w24:string[], "DATA_TYPE"=w23:string[], "PRECISION"=w22:string[])  [unwired: 4 in, 6 out]
      n36 = for {
        tunnel: w59 -> [w89] mode=indexing
        tunnel: [w86] -> w60 mode=indexing
        # "Remove all ?.[  &  [  &  ]"
        n37 = Format Into String(w89) -> (resulting string=w87:string)  [unwired: 3 in, 1 out]
        n38 = Search and Replace String(replace all?=TRUE ("replace all? (F)"), input string=w87, search string="[a-z].\\[+|\\[|\\]") -> (result string=w86:string)  [unwired: 5 in, 3 out]
      }
      n39 = property on="Search User ID" class="CmbBox (strict)"("Strings[]"=w62) -> ()  [unwired: 2 in, 2 out]
      n40 = property on="MCListbox Layout" class="MCListbox (strict)"("ColHdrString"=w52) -> ()  [unwired: 2 in, 2 out]
      n41 = Build Array (concatenate)(w34, w46, w47, w22) -> (w39:string[])
      n42 = Build Array (concatenate)(w35, w42, w43, w24) -> (w41:string[])
      n43 = Build Array (concatenate)(w33, w44, w45, w23) -> (w40:string[])
      "Extra Event From \"Select Foreign Key\" (NA)" <- FALSE ("Extra Event From \"Select Foreign Key Value Changed\"")
      "Record Count" <- 0 ("Record Count")
      "New Record in UI not in DB (NA)" <- FALSE ("New Record in UI not in DB")
      "Output Set Changed" <- FALSE ("Changed")
      "New Layout Id" <- string[] [] ("New Layout Id")
    }
  }
  n44 = while "OutputSet" {
    tunnel: w16 -> [w104]
    tunnel: [w104] -> w15
    tunnel: [w103] -> w14
    tunnel: w12 -> [w106]
    tunnel: w13 -> [w105]
    tunnel: w10 -> [w102]
    tunnel: w9 -> [w101]
    tunnel: w8 -> [w100]
    tunnel: w7 -> [w99]
    tunnel: w6 -> [w98]
    tunnel: w5 -> [w97]
    tunnel: w4 -> [w96]
    tunnel: w3 -> [w95]
    tunnel: w2 -> [w94]
    tunnel: w1 -> [w93]
    stop <- w107 stop-if-true
    n45 = event shown="[12] \"Layout Browse\": Value Change" {
      selector: _ -> [_ _ _ _ _ _ _ _ _ _ _ _ _ _ _ _ _ _ _ _ _ _ _]
      dyn-events: _ -> [_ _ _ _ _ _ _ _ _ _ _ _ _ _ _ _ _ _ _ _ _ _ _]
      timeout: _ -> [_ _ _ _ _ _ _ _ _ _ _ _ _ _ _ _ _ _ _ _ _ _ _]
      tunnel: [_ w110 _ _ _ _ _ _ _ _ _ _ _ _ _ _ _ _ _ _ _ _ _] -> w107
      tunnel: w104 -> [_ _ _ _ w213 _ _ w342 _ w528 w596 _ _ w686 _ _ _ _ _ _ w1058 _ _]
      tunnel: [_ w112 _ _ w129 _ _ w391 _ w511 _ _ _ _ _ _ _ _ _ _ _ _ w1109] -> w103
      tunnel: w106 -> [_ w112 _ _ _ _ _ w341 _ _ _ _ _ _ _ _ _ _ _ _ w1057 _ w1110]
      tunnel: w105 -> [_ _ _ _ _ _ _ w397 _ _ _ _ _ _ _ _ _ _ _ _ _ w1101 w1108]
      tunnel: w102 -> [_ _ _ _ _ _ _ w386 _ w518 _ _ _ w706 _ _ _ _ _ _ _ _ _]
      tunnel: w101 -> [_ _ _ _ _ _ _ _ _ w520 _ _ _ w709 _ _ _ _ _ _ _ _ _]
      tunnel: w100 -> [_ _ _ _ _ _ _ w362 _ _ _ _ _ _ w790 _ _ _ _ _ _ _ _]
      tunnel: w99 -> [_ _ _ _ _ _ _ _ _ _ _ _ _ _ w806 _ _ _ _ _ _ _ _]
      tunnel: w98 -> [_ _ _ _ _ _ _ w348 _ _ _ _ _ _ _ _ _ _ _ _ _ _ _]
      tunnel: w97 -> [_ _ _ _ _ _ _ w347 _ _ _ _ _ _ _ _ _ _ _ _ _ _ _]
      tunnel: w96 -> [_ _ _ _ _ _ _ w346 _ _ _ _ _ _ _ _ _ _ _ _ _ _ _]
      tunnel: w95 -> [_ _ _ _ _ w298 _ _ _ _ _ _ _ _ _ _ _ _ _ _ _ _ _]
      tunnel: w94 -> [_ _ _ _ _ w293 _ _ _ _ _ _ _ _ _ _ _ _ _ _ _ _ _]
      tunnel: w93 -> [_ _ _ _ _ w295 _ _ _ _ _ _ _ _ _ _ _ _ _ _ _ _ _]
      tunnel: [_ _ _ _ w161 _ _ w339 _ w506 _ _ _ w678 _ _ _ _ _ _ _ _ _] -> w92
      event Timeout {
        n46 = event-data() -> ()  [unwired: 1 in, 3 out]
      }
      event "Stop Button": Value Change {
        n47 = event-data() -> ("NewVal"=w111:bool)  [unwired: 1 in, 5 out]
        n48 = flat-sequence {
          tunnel: w111 -> [w113]
          tunnel: [w113] -> w108
          tunnel: [w114] -> w109
          tunnel: w108 -> [w114]
          tunnel: [w116] -> w110
          tunnel: w109 -> [w116]
          frame #0 {
          }
          frame #1 {
            n49 = Wait (ms)(milliseconds to wait=u32 50) -> ()  [unwired: 1 out]
          }
          frame #2 {
            n50 = local write "Stop Button"(FALSE ("Stop Button")) -> ()
          }
        }
      }
      event "------------------------------------        Header EVENTS     ------------------------------------   2": Value Change {
        n51 = event-data() -> ()  [unwired: 1 in, 6 out]
      }
      event "New": Value Change {
        n52 = event-data() -> ()  [unwired: 1 in, 6 out]
        n53 = call "Msgbox - Message Handler.vi"("Short Description (When DB Not Available)"="Create New Output Set", "Description (When DB Not Available)"="All unsaved data will be lost. Do you want to proceed?", "<.?....> Message Code"="<W 541>") -> ("OK Out"=w118:bool)  [unwired: 6 in, 2 out]
        n54 = case shown="True" w118 {
          frame False {
          }
          frame True {
            n55 = property on="Output Set" class="CmbBox (strict)"("Val(Sgnl)"="") -> ()  [unwired: 2 in, 2 out]
          }
        }
      }
      event "Save": Value Change {
        (unwired) string[] ["No.", "Output Type", "Output Type Description", "Layout ID", "Layout Description", "Layout Technical Name", "Output", "Layout File Path", "Output Set", "Inactive"]  # 2014-12-05 08:25 ColHdrs[]
        w144 = 7  # Layout File Path
        w145 = 5  # Layout Technical Name
        w146 = 4  # Layout Decription
        w147 = 3  # Layout ID
        w149 = 3  # Layout ID
        w164 = 6  # Output
        w166 = 1  # Output Type
        w165 = 3  # Layout ID
        w167 = 0  # No.
        w205 = T14[] [enum."[Description]", enum."[Default]", enum."[LastSavedBy]", enum."[LastSavedOn]", enum."[Inactive]"] items=["[PlantId]", "[OutputSetId]", "[Description]", "[Default]", "[CreatedBy]", "[CreatedOn]", "[LastSavedBy]", "[LastSavedOn]", "[Inactive]"]  # [MasterData].[OutputSet] ColNames 2014-11-08 21:03
        # "UPDATE [Config].[Layout]\n   SET [Description] = <Description, nvarchar(30),>\n      ,[LayoutFileName] = <LayoutFileName, nvarchar(50),>\n      ,[LayoutFilePath] = <LayoutFilePath, nvarchar(100),>\n      ,[Inactive] = <Inactive, bit,>\n WHERE <Search Conditions,,>\nGO"
        # "Similar to MasterData.Procedure"
        # "USE [SRTRS]\nGO\n\nINSERT INTO [MasterData].[OutputLayout]\n           ([PlantId]\n           ,[OutputSetId]\n           ,[ItemNo]\n           ,[OutputTypeId]\n           ,[LayoutId]\n           ,[Description]\n           ,[LayoutFileName]\n           ,[LayoutFilePath]\n           ,[Output]\n           ,[Inactive])\n     VALUES\n           (<PlantId, nvarchar(4),>\n           ,<OutputSetId, nvarchar(4),>\n           ,<ItemNo, int,>\n           ,<OutputTypeId, nvarchar(4),>\n           ,<LayoutId, nvarchar(4),>\n           ,<Description, nvarchar(30),>\n           ,<LayoutFileName, nvarchar(50),>\n           ,<LayoutFilePath, nvarchar(100),>\n           ,<Output, bit,>\n           ,<Inactive, bit,>)\nGO"
        # "-- Reinehold Systems Solutions\n--\n-- 2014-11-08 23:03\n--\n\nUSE [SRTRS]\nGO\n\nIF EXISTS (SELECT 1 FROM [MasterData].[OutputSet] WHERE \n\t\t\t[PlantId] = '4070' AND [OutputSetId] = '004' )\nBEGIN\n\nUPDATE [MasterData].[OutputSet]\n   SET [Description] = ''\n      ,[Default] = ''\n      ,[LastSavedBy] = '' \n      ,[LastSavedOn] =  ''\n      ,[Inactive] = '0'\n WHERE [PlantId] = '4070' AND [OutputSetId] = '001'\n\n END\n\n ELSE BEGIN\n INSERT INTO [MasterData].[OutputSet]\n (\t\t[PlantId]\n      ,[OutputSetId]\n      ,[Description]\n      ,[Default]\n      ,[CreatedBy]\n      ,[CreatedOn]\n      ,[LastSavedBy]\n      ,[LastSavedOn]\n      ,[Inactive])\nVALUES ('4070','004','','0','','','','','0')\n\n END"
        # "CAST Leftover Boolean Controls to DB Type\nUPDATE/INSERT DB"
        n56 = event-data() -> ()  [unwired: 1 in, 6 out]
        n57 = local write "Output Set Changed"(FALSE ("Output Set Changed")) -> ()
        n58 = property on="Save" class="Bool"("DisabledEnum"=T5."Disabled and Grayed Out" ("Disabled")) -> ()  [unwired: 2 in, 2 out]
        n59 = global read "Global SRTRS.vi" "Date Time Format"() -> (w201:string)
        n60 = property on="Output Set Header" class="Clust (strict)"() -> ("Value"=w203:T3)  [unwired: 2 in, 2 out]
        n61 = global read "Global SRTRS.vi" "Logon"() -> (w202:T10)
        n62 = Format Date/Time String(time format string (%c)=w201) -> (date/time string=w184:string)  [unwired: 2 in]
        n63 = Unbundle By Name(w203) -> ("Description"=w200:string, "Default"=w199:bool, "Inactive"=w198:bool)
        n64 = Unbundle By Name(w202) -> ("UserID"=w185:string)
        n65 = call "DB - Convert BIT Type.vi"("Boolean"=w198) -> ("BIT (eg Inactive)"=w128:string)  [unwired: 2 in, 2 out]
        n66 = call "DB - Convert BIT Type.vi"("Boolean"=w199) -> ("BIT (eg Inactive)"=w197:string)  [unwired: 2 in, 2 out]
        n67 = Build Array(w200, w197, w185, w184, w128) -> (w186:string[])
        n68 = local read "SRTRS.MasterData.OutputSet"() -> (w206:string)
        n69 = for {
          tunnel: w205 -> [w287] mode=indexing
          tunnel: [w286] -> w204 mode=indexing
          n70 = Format Into String(w287) -> (resulting string=w286:string)  [unwired: 3 in, 1 out]
        }
        n71 = call "DB - Update [Table] Set [ColNames] equ Data.vi"("<Data> (0xFFFE autodetect)"=w186, "[ColumnNames]"=w204) -> ("<Values>"=w192:string)  [unwired: 9 in]
        n72 = call "DB - Split DB.Schema.Table.vi"("DB.Schema.Table"=w206) -> ("DB.Schema.Table"=w207:T15)  [unwired: 10 in]
        n73 = property on="Output Set" class="CmbBox (strict)"() -> ("Value"=w187:T1)  [unwired: 2 in, 2 out]
        n74 = local read "[PlantId]"() -> (w188:string)
        n75 = Build Array (concatenate)(w188, w187, w186, w185, w184) -> (w183:T1[])
        n76 = call "DB - Replace DB.Schema.Table.vi"("DB.Schema.Table"=w207, "string in"="USE [<DB>]\n\nIF EXISTS (SELECT 1 FROM [<Schema>].[<Table>] \nWHERE \t\t[PlantId] = '<P>' AND [OutputSetId] = '<O>' )\n\nBEGIN\nUPDATE [<Schema>].[<Table>]\n   SET <Values>\nWHERE \t\t[PlantId] = '<P>' AND [OutputSetId] = '<O>'\nEND\n\nELSE BEGIN\n INSERT INTO [<Schema>].[<Table>]\n (\t\t[PlantId]\n      ,[OutputSetId]\n      ,[Description]\n      ,[Default]\n      ,[LastSavedBy]\n      ,[LastSavedOn]\n      ,[Inactive]\n       ,[CreatedBy]\n      ,[CreatedOn])\nVALUES (<Values2>)\n\n END") -> ("string out"=w208:string)  [unwired: 8 in, 1 out]
        n77 = Search and Replace String(replace all?=TRUE ("replace all? (F)"), input string=w208, search string="<P>", replace string=w188) -> (result string=w210:string)  [unwired: 4 in, 3 out]
        n78 = call "DB - Array to Values.vi"("Array (0xFFFE autodetect)"=w183) -> ("<Values>"=w189:string)  [unwired: 10 in]
        n79 = disable-structure shown="Disabled" {
          frame Disabled {
            n80 = call "Msgbox - Format Message.vi"("Message Code\n2014-10-01"=Message_Code_-_Enum."<DB><I 300>" ("Message Code\n2014-10-01")) -> ("Message"=w285:string)  [unwired: 9 in, 1 out]
            n81 = call "Msgbox UI.vi"("[MessageType]"=w285) -> ()  [unwired: 8 in, 3 out]
          }
          frame Enabled {
          }
        }
        n82 = Search and Replace String(replace all?=TRUE ("replace all? (F)"), input string=w210, search string="<O>", replace string=w187) -> (result string=w196:string)  [unwired: 4 in, 3 out]
        n83 = Search and Replace String(input string=w196, search string="<Values>", replace string=w192) -> (result string=w191:string)  [unwired: 5 in, 3 out]
        n84 = Search and Replace String(input string=w191, search string="<Values2>", replace string=w189) -> (result string=w162:string)  [unwired: 5 in, 3 out]
        n85 = call-poly <vilib>:"DB Tools Execute Query.vi"("SQL query"=w162, "connection reference"=w213) -> ("error out"=w181:errorcluster, "recordset reference"=w182:T16)  [unwired: 6 in]
        n86 = call-poly <vilib>:"DB Tools Free Object.vi"("error in (no error)"=w181, "recordset reference"=w182) -> ("error out"=w163:errorcluster, "connection reference"=w140:T12)  [unwired: 8 in]
        n87 = property on="MCListbox Layout" class="MCListbox (strict)"() -> ("ItemNames"=w158:string[][])  [unwired: 2 in, 2 out]
        n88 = for {
          shift-right: [w279] -> w137
          shift-left: "" -> [w280]
          tunnel: w158 -> [w276] mode=indexing
          tunnel: w167 -> [w275]
          tunnel: w166 -> [w274]
          tunnel: w165 -> [w273]
          tunnel: w164 -> [w269]
          tunnel: w128 -> [w260]
          i -> [w267]
          w277 = "<O>"  # [OutputSetId]
          w278 = "<P>"  # [PlantId]
          n89 = Index Array(array=w276, index #1=w275, index #2=w274, index #3=w273, index #4=w269) -> (element #1=w272:string, element #2=w271:string, element #3=w268:string, element #4=w270:string)
          n90 = Equal To 0?(x=w267) -> (x = 0?=w266:bool)
          n91 = Build Array(w278, w277, w272, w271, w268, w270, w260) -> (w262:string[])
          n92 = Array To Spreadsheet String(delimiter (Tab)="','", array=w262, 3:"" ("format string")) -> ()  [unwired: 1 out]
          n93 = Select(t="(" ("string"), s=w266, f=",(" ("string")) -> (s? t:f=w265:string)
          n94 = call "DB - Array to Values.vi"("Array (0xFFFE autodetect)"=w262) -> ("<Values>"=w261:string)  [unwired: 10 in]
          n95 = Concatenate Strings(w280, w265, w261, ")" ("string")) -> (w279:string)
        }
        n96 = local read "SRTRS.MasterData.OutputLayout"() -> (w176:string)
        n97 = Array Size(array=w158) -> (size(s)=w157:i32[])
        n98 = call "DB - Split DB.Schema.Table.vi"("DB.Schema.Table"=w176) -> ("DB.Schema.Table"=w175:T15)  [unwired: 10 in]
        n99 = Index Array(array=w157) -> (element=w156:i32)  [unwired: 1 in]
        n100 = call "DB - Replace DB.Schema.Table.vi"("DB.Schema.Table"=w175, "string in"="USE [<DB>]\n\nIF EXISTS (SELECT 1 FROM [<Schema>].[<Table>] \nWHERE \t\t[PlantId] = '<P>' AND [OutputSetId] = '<O>'  )\nBEGIN\nDELETE FROM [<Schema>].[<Table>]\nWHERE \t\t\t[PlantId] = '<P>' AND [OutputSetId] = '<O>' \n\nEND\n\nINSERT INTO [MasterData].[OutputLayout]\n (\t   \t[PlantId]\n      ,[OutputSetId]\n      ,[ItemNo]\n      ,[OutputTypeId]\n      ,[LayoutId]\n      ,[Output]\n      ,[Inactive]\n)\n VALUES \n(<Values>)\n\n") -> ("string out"=w168:string)  [unwired: 8 in, 1 out]
        n101 = local read "[PlantId]"() -> (w160:string)
        n102 = Search and Replace String(input string=w168, search string="(<Values>)", replace string=w137) -> (result string=w169:string)  [unwired: 5 in, 3 out]
        n103 = property on="Output Set" class="CmbBox (strict)"() -> ("Value"=w159:T1)  [unwired: 2 in, 2 out]
        n104 = Search and Replace String(replace all?=TRUE ("replace all? (F)"), input string=w169, search string="<P>", replace string=w160) -> (result string=w174:string)  [unwired: 4 in, 3 out]
        n105 = Search and Replace String(replace all?=TRUE ("replace all? (F)"), input string=w174, search string="<O>", replace string=w159) -> (result string=w152:string)  [unwired: 4 in, 3 out]
        n106 = Search and Replace String(replace all?=TRUE ("replace all? (F)"), input string=w152, search string="<L>") -> (result string=w151:string)  [unwired: 5 in, 3 out]
        n107 = case shown="1, Default" w156 {
          tunnel: w163 -> [w253 w257]
          tunnel: [w253 w256] -> w139
          tunnel: w140 -> [_ w255]
          tunnel: w151 -> [_ w254]
          frame 0 {
            # "No Data. No need to INSERT to [Output].[Layout]"
          }
          frame 1, Default {
            n108 = call-poly <vilib>:"DB Tools Execute Query.vi"("error in (no error)"=w257, "SQL query"=w254, "connection reference"=w255) -> ("error out"=w259:errorcluster, "recordset reference"=w258:T16)  [unwired: 5 in]
            n109 = call-poly <vilib>:"DB Tools Free Object.vi"("error in (no error)"=w259, "recordset reference"=w258) -> ("error out"=w256:errorcluster)  [unwired: 8 in, 1 out]
          }
        }
        "DB" <- w139
        n110 = local read "New Layout Id"() -> (w143:string[])
        n111 = property on="MCListbox Layout" class="MCListbox (strict)"() -> ("ItemNames"=w136:string[][])  [unwired: 2 in, 2 out]
        n112 = global write "Global SRTRS.vi" "DB Error"(w139) -> ()
        n113 = local read "SRTRS.MasterData.Layout"() -> (w150:string)
        n114 = Array Size(array=w136) -> (size(s)=w135:i32[])
        n115 = Index Array(array=w136, index (col)=w149) -> (element=w148:string[])  [unwired: 1 in]
        n116 = Index Array(array=w135) -> (element=w134:i32)  [unwired: 1 in]
        n117 = for {
          tunnel: w143 -> [w251] mode=indexing
          tunnel: w148 -> [w252]
          tunnel: [w250] -> w131 mode=indexing if=w249
          n118 = Search 1D Array(1D array=w252, element=w251) -> (index of element=w250:i32)  [unwired: 1 in]
          n119 = Greater Or Equal To 0?(x=w250) -> (x >= 0?=w249:bool)
        }
        n120 = for {
          N: w134 -> [_]
          tunnel: [w214] -> w132 mode=indexing
          i -> [w214]
        }
        n121 = call "DB - Split DB.Schema.Table.vi"("DB.Schema.Table"=w150) -> ("DB.Schema.Table"=w142:T15)  [unwired: 10 in]
        n122 = Select(t=w132, s="UPDATE ALL LayoutId", f=w131) -> (s? t:f=w130:i32[])
        n123 = for {
          tunnel: w136 -> [w248]
          tunnel: w130 -> [w247] mode=indexing
          tunnel: w147 -> [w245]
          tunnel: w146 -> [w244]
          tunnel: w145 -> [w243]
          tunnel: w144 -> [w242]
          tunnel: w142 -> [w236]
          tunnel: "USE [<DB>]\n\nUPDATE [<Schema>].[<Table>]\nSET  (<Values>)\nWHERE [LayoutId] = '<L>'\n\n" -> [w235]
          tunnel: w140 -> [w226]
          tunnel: [w223] -> w138 mode=indexing
          shift-right: [w224] -> w129
          shift-left: w139 -> [w225]
          tunnel: w128 -> [w222]
          n124 = Index Array(array=w248, index (row)=w247) -> (element=w246:string[])  [unwired: 1 in]
          n125 = Index Array(array=w246, index #1=w245, index #2=w244, index #3=w243, index #4=w242) -> (element #1=w232:string, element #2=w241:string, element #3=w240:string, element #4=w239:string)
          n126 = call "DB - Replace DB.Schema.Table.vi"("DB.Schema.Table"=w236, "string in"=w235) -> ("string out"=w238:string)  [unwired: 8 in, 1 out]
          n127 = Build Array(w241, w240, w239, w222) -> (w230:string[])
          n128 = call "DB - Update [Table] Set [ColNames] equ Data.vi"("<Data> (0xFFFE autodetect)"=w230, "[ColumnNames]"=string[] ["[Description]", "[LayoutFileName]", "[LayoutFilePath]", "[Inactive]"]) -> ("<Values>"=w229:string)  [unwired: 9 in]
          n129 = Search and Replace String(input string=w238, search string="(<Values>)", replace string=w229) -> (result string=w234:string)  [unwired: 5 in, 3 out]
          n130 = Search and Replace String(input string=w234, search string="<L>", replace string=w232) -> (result string=w223:string)  [unwired: 5 in, 3 out]
          n131 = call-poly <vilib>:"DB Tools Execute Query.vi"("error in (no error)"=w225, "SQL query"=w223, "connection reference"=w226) -> ("error out"=w227:errorcluster, "recordset reference"=w228:T16)  [unwired: 5 in]
          n132 = call-poly <vilib>:"DB Tools Free Object.vi"("error in (no error)"=w227, "recordset reference"=w228) -> ("error out"=w224:errorcluster)  [unwired: 8 in, 1 out]
        }
        n133 = case shown="Error" w129 {
          tunnel: ["Output Set Saved" ("Short Description (When DB Not Available)") "Ouput Set Save Failed" ("Short Description (When DB Not Available)")] -> w127
          tunnel: [" output set details saved." ("Short Description (When DB Not Available)") " output set details cannot be saved." ("Short Description (When DB Not Available)")] -> w126
          tunnel: ["<I 543>" ("Short Description (When DB Not Available)") "<E 548>" ("Short Description (When DB Not Available)")] -> w124
          frame No Error {
            n134 = local write "New Layout Id"(string[] [] ("New Layout Id")) -> ()
          }
          frame Error {
          }
        }
        n135 = property on="Output Set" class="CmbBox (strict)"() -> ("Value"=w125:T1)  [unwired: 2 in, 2 out]
        n136 = Build Array (concatenate)(w162, w151, w138) -> (w161:string[])
        n137 = call "Msgbox - Message Handler.vi"("Short Description (When DB Not Available)"=w127, "Description (When DB Not Available)"=w126, "Pre-Description"=w125, "<.?....> Message Code"=w124) -> ("MHandler Error"=w123:errorcluster)  [unwired: 5 in, 2 out]
        n138 = local write "MHandler"(w123) -> ()
      }
      event Value Change {
        n139 = event-data() -> ("CtlRef"=w297:refnum<vi>)  [unwired: 1 in, 5 out]
        n140 = property class="Str"(reference=w297) -> (reference out=w290:refnum<vi>, "Label.Text"=w296:string, "Value"=w291:string)  [unwired: 1 in, 1 out]
        n141 = Search 1D Array(1D array=w298, element=w296) -> (index of element=w292:i32)  [unwired: 1 in]
        n142 = local write "Output Set Changed"(TRUE ("Output Set Changed")) -> ()
        n143 = property on="Save" class="Bool"("DisabledEnum"=T5."Enabled" ("Disabled")) -> ()  [unwired: 2 in, 2 out]
        n144 = Index Array(array=w295, index=w292) -> (element=w294:string)
        n145 = case "CAST INTO Correct TYPE and PRECISION" shown="\"nvarchar\", Default" w294 {
          tunnel: w293 -> [w304 _]
          tunnel: w292 -> [w303 _]
          tunnel: w291 -> [w302 _]
          tunnel: w290 -> [w300 _]
          frame "nvarchar", Default {
            n146 = Index Array(array=w304, index=w303) -> (element=w305:string)
            n147 = Decimal String To Number(string=w305) -> (number=w301:i32)  [unwired: 2 in, 1 out]
            "Precision" <- w301
            n148 = String Subset(string=w302, length (rest)=w301) -> (substring=w299:string)  [unwired: 1 in]
            n149 = property class="Str"(reference=w300, "Value"=w299) -> ()  [unwired: 1 in, 2 out]
          }
          frame "" {
            # "NA"
          }
        }
      }
      event Value Change {
        n150 = event-data() -> ("CtlRef"=w311:refnum<vi>, "NewVal"=w309:bool)  [unwired: 1 in, 4 out]
        n151 = property class="Bool (strict)"(reference=w311) -> (reference out=w308:refnum<vi>, "Label.Text"=w310:string)  [unwired: 1 in, 1 out]
        n152 = property on="Output Set" class="CmbBox (strict)"() -> ("Value"=w307:T1)  [unwired: 2 in, 2 out]
        n153 = Empty String/Path?(string/path=w307) -> (empty?=w306:bool)
        n154 = case shown="False" w306 {
          tunnel: w310 -> [w316 _]
          tunnel: w309 -> [w315 _]
          tunnel: w308 -> [w314 _]
          tunnel: w307 -> [w312 _]
          frame False {
            # "Output Set NOT empty"
            n155 = case shown="\"Inactive\"" w316 {
              tunnel: w315 -> [_ w323]
              tunnel: w314 -> [_ w322]
              tunnel: [TRUE ("OK Out") w321] -> w313
              tunnel: w312 -> [_ w320]
              frame "Output Set", Default {
              }
              frame "Inactive" {
                n156 = case shown="True" w323 {
                  tunnel: w322 -> [_ w328]
                  tunnel: [TRUE ("OK Out") w327] -> w321
                  tunnel: w320 -> [_ w326]
                  frame False {
                  }
                  frame True {
                    n157 = call "Msgbox - Message Handler.vi"("Short Description (When DB Not Available)"="Inactive Output Set", "Description (When DB Not Available)"=" output set cannot be used after inactive. Do you wish to proceed?", "Pre-Description"=w326, "<.?....> Message Code"="<W 544>") -> ("MHandler Error"=w325:errorcluster, "OK Out"=w327:bool)  [unwired: 5 in, 1 out]
                    n158 = case shown="True" w327 {
                      selector: w327 -> [_ w332]
                      tunnel: w328 -> [_ w333]
                      frame False {
                      }
                      frame True {
                        n159 = property class="Bool (strict)"(reference=w333, "Value"=w332) -> ()  [unwired: 1 in, 2 out]
                      }
                    }
                    n160 = local write "MHandler"(w325) -> ()
                  }
                }
              }
            }
            n161 = case shown="True" w313 {
              frame False {
              }
              frame True {
                n162 = local write "Output Set Changed"(TRUE ("Output Set Changed")) -> ()
                n163 = property on="Save" class="Bool"("DisabledEnum"=T5."Enabled" ("Disabled")) -> ()  [unwired: 2 in, 2 out]
              }
            }
          }
          frame True {
            # "Output Set empty"
          }
        }
      }
      event Value Change {
        w359 = 0 ("index (row)")
        w393 = T9 {"Row"=-1, "Column"=-2}  # Col Hdr
        w402 = T9 {"Row"=-2, "Column"=-2}  # Invalid ALL
        # "For Combine to work,\nAssumption is that the duplicated\ncolumn names across the tables\nshare the same Data Type and Precision"
        # "Show [Inactive] also"
        # ",FORMAT(b.[LastCalibDate], 'yyyy-MM-dd')\n  ,FORMAT(b.[NextCalibDate], 'yyyy-MM-dd')"
        # "-- Reinehold Systems Solutions\n-- \n-- 2014-11-10 13:04\n--\n-- \nUSE [SRTRS]\n\nSELECT\n    b.[ItemNo]\n    ,a.[OutputSetId] \n    ,a.[Description]\n    ,a.[Default]\n    ,a.[Inactive]\n    ,b.[OutputTypeId]\n    ,c.[ShortDescription] AS [OutputType Description] \n    ,b.[Output]\n    ,b.[Inactive]\n    ,b.[LayoutId]\n    ,d.[Description] AS [Layout Description]\n    ,d.[LayoutFileName]\n    ,d.[LayoutFilePath]\nFROM [MasterData].[OutputSet] as a\nJOIN [MasterData].[OutputLayout] as b\nON a.[PlantId] = b.[PlantId] AND\n       a.[OutputSetId] = b.[OutputSetId]\nLEFT JOIN [Config].[OutputType] as c\nON b.[OutputTypeId] = c.[OutputTypeId] \n\nLEFT JOIN [Config].[Layout] as d\nON b.[LayoutId] = d.[LayoutId]\n\nWHERE\na.[PlantId] = '4070' AND\na.[OutputSetId] = '001'\n\nORDER BY [ItemNo] ASC"
        # "Only SRTRS.MasterData.OutputType checked"
        # "Only DB Column Names \nupdated to MCListbox Col0"
        # "SELECT Table & Column Information FROM DB\nSELECT * FROM DB"
        n164 = event-data() -> ()  [unwired: 1 in, 6 out]
        n165 = local read "SRTRS.Config.OutputType"() -> (w343:string)
        n166 = local read "SRTRS.MasterData.OutputSet"() -> (w345:string)
        n167 = local read "SRTRS.MasterData.OutputLayout"() -> (w344:string)
        n168 = local read "SRTRS.MasterData.Layout"() -> (w338:string)
        n169 = call "DB - Split DB.Schema.Table.vi"("DB.Schema.Table"=w338) -> ("DB.Schema.Table"=w337:T15)  [unwired: 10 in]
        n170 = call "DB - Split DB.Schema.Table.vi"("DB.Schema.Table"=w344) -> ("DB.Schema.Table"=w373:T15)  [unwired: 10 in]
        n171 = call "DB - Split DB.Schema.Table.vi"("DB.Schema.Table"=w343) -> ("DB.Schema.Table"=w372:T15)  [unwired: 10 in]
        n172 = call "DB - Split DB.Schema.Table.vi"("DB.Schema.Table"=w345) -> ("DB.Schema.Table"=w378:T15)  [unwired: 10 in]
        n173 = call "DB - Replace DB.Schema.Table.vi"("DB.Schema.Table 4"=w337, "DB.Schema.Table 3"=w372, "DB.Schema.Table 2"=w373, "DB.Schema.Table"=w378, "string in"="USE [<DB>]\n\nSELECT\n     b.[ItemNo]\n    ,a.[OutputSetId] \n    ,a.[Description]\n    ,a.[Default]\n    ,a.[Inactive]\n    ,b.[OutputTypeId]\n    ,c.[ShortDescription] AS [OutputType Description] \n    ,b.[Output]\n    ,b.[Inactive]\n    ,b.[LayoutId]\n    ,d.[Description] AS [Layout Description]\n    ,d.[LayoutFileName]\n    ,d.[LayoutFilePath]\nFROM [<Schema>].[<Table>] as a\nJOIN [<Schema2>].[<Table2>] as b\nON a.[PlantId] = b.[PlantId] AND\n       a.[OutputSetId] = b.[OutputSetId]\nLEFT JOIN [<Schema3>].[<Table3>] as c\nON b.[OutputTypeId] = c.[OutputTypeId] \nLEFT JOIN [<Schema4>].[<Table4>] as d\nON b.[LayoutId] = d.[LayoutId]\nWHERE\na.[PlantId] = '<P>' AND\na.[OutputSetId] = '<O>' \nORDER BY [ItemNo] ASC\n\n") -> ("string out"=w369:string)  [unwired: 5 in, 1 out]
        n174 = property on="Output Set" class="CmbBox (strict)"() -> ("Text.Text"=w364:string)  [unwired: 2 in, 2 out]
        n175 = Search and Replace String(input string=w369, search string="<P>", replace string="[PlantId]") -> (result string=w368:string)  [unwired: 5 in, 3 out]
        n176 = Search and Replace String(input string=w368, search string="<O>", replace string=w364) -> (result string=w340:string)  [unwired: 5 in, 3 out]
        n177 = call-poly <vilib>:"DB Tools Execute Query.vi"("error in (no error)"=w341, "SQL query"=w340, "connection reference"=w342) -> ("error out"=w385:errorcluster, "recordset reference"=w384:T16)  [unwired: 5 in]
        n178 = call-poly <vilib>:"DB Tools Fetch Recordset Data.vi"("error in (no error)"=w385, "recordset reference"=w384) -> ("error out"=w380:errorcluster, "recordset data"=w383:variant[][], "recordset reference out"=w381:T16)  [unwired: 3 in]
        n179 = xnode "Database Variant To Data"("database variant"=w383, "type"=string[][] []) -> ("data"=w360:string[][])  [unwired: 1 in, 1 out]
        n180 = call-poly <vilib>:"DB Tools Free Object.vi"("error in (no error)"=w380, "recordset reference"=w381) -> ("error out"=w363:errorcluster)  [unwired: 8 in, 1 out]
        "Property Node" <- w363
        n181 = for {
          tunnel: w360 -> [w483]
          tunnel: w386 -> [w475] mode=indexing
          tunnel: [w482] -> w388 mode=indexing
          tunnel: w348 -> [w481]
          tunnel: w347 -> [w480]
          tunnel: [w479] -> w370 mode=indexing
          tunnel: w346 -> [w477]
          tunnel: [w476] -> w374 mode=indexing
          tunnel: w362 -> [w474] mode=indexing
          n182 = Index Array(array=w483, index (col)=w474) -> (element=w482:string[])  [unwired: 1 in]
          n183 = Search 1D Array "Match Col Hdrs[]\nData Type"(1D array=w481, element=w475) -> (index of element=w478:i32)  [unwired: 1 in]
          n184 = Index Array(array=w480, index=w478) -> (element=w479:string)
          n185 = Index Array(array=w477, index=w478) -> (element=w476:string)
        }
        "Col Hdrs[] DB Data Type" <- w370
        "Col Hdrs[] DB Precision" <- w374
        n186 = Index Array "Header Information"(array=w360, index (row) #1=w359, index (col) #1=DB_-_Master_Data_Layout_Enum."a.[Description]" ("2014-11-07 13:45\nMaster Data Layout"), index (row) #2=w359, index (col) #2=DB_-_Master_Data_Layout_Enum."a.[Default]" ("2014-11-07 13:45\nMaster Data Layout"), index (row) #3=w359, index (col) #3=DB_-_Master_Data_Layout_Enum."a.[Inactive]" ("2014-11-07 13:45\nMaster Data Layout")) -> (element #1=w351:string, element #2=w355:string, element #3=w354:string)
        n187 = call "DB - Convert BIT Type.vi"("BIT Type (eg Inactive)"=w355) -> ("Boolean"=w350:bool)  [unwired: 2 in, 2 out]
        n188 = call "DB - Convert BIT Type.vi"("BIT Type (eg Inactive)"=w354) -> ("Boolean"=w349:bool)  [unwired: 2 in, 2 out]
        n189 = Transpose 2D Array(2D array=w388) -> (transposed array=w371:string[][])
        n190 = property on="Header" class="Clust (strict)"() -> ("Value"=w352:T17)  [unwired: 2 in, 2 out]
        n191 = Bundle By Name(cluster=w352, "Description"=w351, "Default"=w350, "Inactive"=w349) -> (w353:T17)
        n192 = for "Convert DB Data Type to Strings" {
          tunnel: w371 -> [w416] mode=indexing
          tunnel: w370 -> [w415]
          tunnel: [w414] -> w361 mode=indexing
          # "Row"
          n193 = for {
            tunnel: w416 -> [w418] mode=indexing
            tunnel: w415 -> [w419] mode=indexing
            tunnel: [w417] -> w414 mode=indexing
            # "Column"
            n194 = case shown="\"bit\"" w419 {
              tunnel: w418 -> [w420 w422 w426]
              tunnel: [w420 w421 w425] -> w417
              frame "False", Default {
              }
              frame "bit" {
                n195 = case shown="\"-1\", Default" w422 {
                  selector: w422 -> [_ w424]
                  tunnel: ["1" w424] -> w421
                  frame "-1", Default {
                  }
                  frame "0" {
                  }
                }
              }
              frame "datetime", "datetime2" {
                # "SQL Server Default"
                n196 = Equal?(x=w426, y="1900-01-01") -> (x = y?=w428:bool)
                n197 = Select(t="", s=w428, f=w426) -> (s? t:f=w425:string)
              }
            }
          }
        }
        n198 = property on="Header" class="Clust (strict)"("Value"=w353) -> ()  [unwired: 2 in, 2 out]
        n199 = local read "CellBG Unused Cells"() -> (w334:u32)
        n200 = local read "CellBG ColHdrs"() -> (w336:u32)
        n201 = local read "CellBG New Cells"() -> (w335:u32)
        n202 = flat-sequence {
          tunnel: w361 -> [w413]
          frame #0 {
            # "Reinit contents when new Record is loaded"
            n203 = Array Size(array=w413) -> (size(s)=w412:i32[])
            n204 = local write "Current Record"(0 ("Current Record")) -> ()
            n205 = Index Array(array=w412) -> (element=w404:i32)  [unwired: 1 in]
            n206 = local write "Editing Layout Details in New Record"(FALSE ("Editing Layout Details in New Record")) -> ()
            n207 = Increment(x=w404) -> (x+1=w410:i32)
            n208 = local write "All Mandatory Fields Filled"(FALSE ("All Mandatory Fields Filled")) -> ()
            n209 = local write "Output Set Changed"(FALSE ("Output Set Changed")) -> ()
            n210 = local write "Record Count"(w404) -> ()
            n211 = local write "Item Number"(w410) -> ()
            n212 = property on="MCListbox Layout" class="MCListbox (strict)"("Value"=w404) -> ()  [unwired: 2 in, 2 out]
            n213 = property on="New" class="Bool"("DisabledEnum"=T5."Enabled" ("Disabled")) -> ()  [unwired: 2 in, 2 out]
            n214 = invoke on="Layout Details Cluster" class="Clust (strict)" method="Reinit To Default"() -> ()  [unwired: 3 in, 3 out]
            n215 = property on="Save" class="Bool"("DisabledEnum"=T5."Disabled and Grayed Out" ("Disabled")) -> ()  [unwired: 2 in, 2 out]
            n216 = property on="Delete" class="Bool"("DisabledEnum"=T5."Disabled and Grayed Out" ("Disabled")) -> ()  [unwired: 2 in, 2 out]
          }
        }
        n217 = Index Array(array=w361, index (col)=0 ("disabled index (col)")) -> (element=w376:string[])  [unwired: 1 in]
        n218 = property on="Property Node" class="MCListbox (strict)"(reference=w397, error in=w363, "ItemNames"=w361, "ActiveCell"=w402, "CellBG"=w334, "CellFontBold"=FALSE ("Active Cell:Cell Font:Bold"), "NumCols"="# of Columns", "NumRows"="# of Rows") -> (reference out=w396:refnum<vi>, error out=w395:errorcluster)
        n219 = property on="Search User ID" class="CmbBox (strict)"("Strings[]"=w376) -> ()  [unwired: 2 in, 2 out]
        n220 = property on="Property Node" class="MCListbox (strict)"(reference=w396, error in=w395, "ActiveCell"=w393, "CellBG"=w336) -> (reference out=w389:refnum<vi>, error out=w394:errorcluster)
        n221 = for {
          N: 0 -> [_]
          tunnel: w335 -> [w500]
          shift-right: [w504] -> w401
          shift-left: w394 -> [w505]
          shift-right: [w498] -> w399
          shift-left: w389 -> [w499]
          i -> [w503]
          # "Color Each Row"
          n222 = Bundle(w503, -2) -> (w501:cluster{i32, i32})  [unwired: 1 in]
          n223 = property on="Property Node" class="MCListbox (strict)"(reference=w499, error in=w505, "ActiveCell"=w501, "CellBG"=w500) -> (reference out=w498:refnum<vi>, error out=w504:errorcluster)
        }
        n224 = for {
          N: 10 -> [_]
          tunnel: w334 -> [w493]
          tunnel: "# of Columns" -> [w491]
          shift-right: [w496] -> w391
          shift-left: w401 -> [w497]
          shift-right: [w488] -> w390
          shift-left: w399 -> [w489]
          i -> [w492]
          # "Invalid Leftover Columns"
          n225 = Add(x=w491, y=w492) -> (x+y=w490:i32)
          n226 = Bundle(-2, w490) -> (w495:cluster{i32, i32})  [unwired: 1 in]
          n227 = property on="Property Node" class="MCListbox (strict)"(reference=w489, error in=w497, "ActiveCell"=w495, "CellBG"=w493) -> (reference out=w488:refnum<vi>, error out=w496:errorcluster)
        }
        n228 = case shown="No Error" w391 {
          tunnel: w390 -> [_ w487]
          frame No Error {
          }
          frame Error {
            n229 = property on="Property Node" class="MCListbox (strict)"(reference=w487, "Value"=-1, "ItemNames"=string[][] [] ("Item Names")) -> (error out=w484:errorcluster)  [unwired: 1 in, 1 out]
            n230 = local write "Property Node"(w484) -> ()
          }
        }
        n231 = Build Array(w340) -> (w339:string[])
      }
      event "------------------------------------        Layout Details EVENTS     ------------------------------------": Value Change {
        # "DUMMY EVENT"
        n232 = event-data() -> ()  [unwired: 1 in, 6 out]
      }
      event Mouse Down? {
        # "Query for Values of OutputSetId OR OutputTypeId \nto populate their respective ComboBox"
        n233 = event-data() -> ("CtlRef"=w521:refnum<vi>)  [unwired: 1 in, 7 out]
        n234 = property class="CmbBox (strict)"(reference=w521) -> ("Label.Text"=w510:string)  [unwired: 1 in, 2 out]
        n235 = Search 1D Array(1D array=w520, element=w510) -> (index of element=w519:i32)  [unwired: 1 in]
        n236 = Index Array(array=w518, index=w519) -> (element=w508:string)
        n237 = case shown="\"OutputTypeId\"" w508 {
          tunnel: [w535 w537 w539] -> w513
          tunnel: ["USE [<DB>]\n\nSELECT [<A>]\nFROM [<Schema>].[<Table>]\n\nWHERE [PlantId] = '<P>' AND [Inactive] = '0'\nGROUP BY [<A>]\nORDER BY [<A>] ASC\n" "USE [<DB>]\n\nSELECT [<A>]\nFROM [<Schema>].[<Table>]\n\nWHERE [Inactive] = '0'\nGROUP BY [<A>]\nORDER BY [<A>] ASC\n" "USE [<DB>]\n\nSELECT [<A>]\nFROM [<Schema>].[<Table>]\n\nWHERE [Inactive] = '0'\nGROUP BY [<A>]\nORDER BY [<A>] ASC\n"] -> w512
          frame "OutputSetId", Default {
            n238 = local read "SRTRS.MasterData.OutputSet"() -> (w535:string)
          }
          frame "OutputTypeId" {
            n239 = local read "SRTRS.Config.OutputType"() -> (w537:string)
          }
          frame "LayoutId" {
            n240 = local read "SRTRS.MasterData.Layout"() -> (w539:string)
          }
        }
        n241 = call "DB - Split DB.Schema.Table.vi"("DB.Schema.Table"=w513) -> ("DB.Schema.Table"=w527:T15)  [unwired: 10 in]
        n242 = call "DB - Replace DB.Schema.Table.vi"("DB.Schema.Table"=w527, "string in"=w512) -> ("string out"=w517:string)  [unwired: 8 in, 1 out]
        n243 = local read "[PlantId]"() -> (w509:string)
        n244 = Search and Replace String(replace all?=TRUE ("replace all? (F)"), input string=w517, search string="<A>", replace string=w508) -> (result string=w516:string)  [unwired: 4 in, 3 out]
        n245 = Search and Replace String(input string=w516, search string="<P>", replace string=w509) -> (result string=w507:string)  [unwired: 5 in, 3 out]
        n246 = call-poly <vilib>:"DB Tools Execute Query.vi"("SQL query"=w507, "connection reference"=w528) -> ("error out"=w534:errorcluster, "recordset reference"=w533:T16)  [unwired: 6 in]
        n247 = call-poly <vilib>:"DB Tools Fetch Recordset Data.vi"("error in (no error)"=w534, "recordset reference"=w533) -> ("error out"=w529:errorcluster, "recordset data"=w532:variant[][], "recordset reference out"=w530:T16)  [unwired: 3 in]
        n248 = xnode "Database Variant To Data"("database variant"=w532, "type"=string[][] []) -> ("data"=w525:string[][])  [unwired: 1 in, 1 out]
        n249 = call-poly <vilib>:"DB Tools Free Object.vi"("error in (no error)"=w529, "recordset reference"=w530) -> ("error out"=w511:errorcluster)  [unwired: 8 in, 1 out]
        n250 = Index Array(array=w525, index (col)=0 ("disabled index (col)")) -> (element=w523:string[])  [unwired: 1 in]
        n251 = local write "DB"(w511) -> ()
        n252 = property class="CmbBox (strict)"(reference=w521, error in=w511, "Strings[]"=w523) -> (error out=w522:errorcluster)  [unwired: 1 out]
        n253 = global write "Global SRTRS.vi" "DB Error"(w511) -> ()
        n254 = local write "Property Node"(w522) -> ()
        n255 = Build Array(w507) -> (w506:string[])
        n256 = event-data() -> ()  [unwired: 2 in, 1 out]
      }
      event "New Layout ID": Value Change {
        w594 = 0 ("index (row)")
        # "USE [SRTRS]\n\n\nINSERT INTO [Config].[Layout] ([Inactive]) VALUES ('0')"
        n257 = event-data() -> ()  [unwired: 1 in, 6 out]
        n258 = local read "SRTRS.MasterData.Layout"() -> (w599:string)
        n259 = call "DB - Split DB.Schema.Table.vi"("DB.Schema.Table"=w599) -> ("DB.Schema.Table"=w600:T15)  [unwired: 10 in]
        n260 = call "DB - Replace DB.Schema.Table.vi"("DB.Schema.Table"=w600, "string in"="USE [<DB>]\nDECLARE @value as int\nEXEC GetNewLayoutID  @layoutID = @value OUTPUT") -> ("string out"=w597:string)  [unwired: 8 in, 1 out]
        n261 = call "DB - T-SQL Query.vi"("T-SQL"=w597, "connection reference"=w596) -> ("error out"=w591:errorcluster, "2D data"=w595:string[][])  [unwired: 7 in, 1 out]
        n262 = Index Array(array=w595, index (row)=w594, index (col)=w594) -> (element=w587:string)
        n263 = local read "New Layout Id"() -> (w585:string[])
        n264 = local write "DB"(w591) -> ()
        n265 = Empty String/Path?(string/path=w587) -> (empty?=w593:bool)
        n266 = Not(x=w593) -> (.not. x?=w592:bool)
        n267 = Unbundle By Name(w591) -> ("status"=w590:bool)
        n268 = Build Array (concatenate)(w585, w587) -> (w586:string[])
        n269 = Not(x=w590) -> (.not. x?=w589:bool)
        n270 = local write "New Layout Id"(w586) -> ()
        n271 = And(x=w589, y=w592) -> (x .and. y?=w588:bool)
        n272 = case shown="True" w588 {
          tunnel: w587 -> [_ w601]
          frame False {
          }
          frame True {
            n273 = property on="Layout Description" class="Str"("DisabledEnum"=T5."Enabled" ("Disabled"), "Text.BG Color"=u32 16777215) -> ()  [unwired: 2 in, 2 out]
            n274 = property on="Layout ID" class="CmbBox (strict)"("Value"=w601) -> ()  [unwired: 2 in, 2 out]
          }
        }
      }
      event "Item Number": Value Change {
        # "User Changes Item No\nCheck for valid values then set MCListBox EVENT"
        n275 = event-data() -> ("NewVal"=w604:i32)  [unwired: 1 in, 5 out]
        n276 = flat-sequence {
          tunnel: w604 -> [w608]
          frame #0 {
            # "Upper Limit is ItemNames  #Rows + 1\nLower Limit is the smaller of 1 and #Rows"
            # "ItemNo Value Change EVENT\nThis Sequence Controls the MCListoBox Value to show\nThe other Sequence will be in the MCListBox Value Change EVENT which sets the ItemNo Value"
            n277 = property on="MCListbox Layout" class="MCListbox (strict)"() -> ("ItemNames"=w613:string[][])  [unwired: 2 in, 2 out]
            n278 = Array Size(array=w613) -> (size(s)=w612:i32[])
            n279 = Index Array(array=w612) -> (element=w609:i32)  [unwired: 1 in]
            n280 = Max & Min(x=w609, y=1) -> (min(x,y)=w610:i32)  [unwired: 1 out]
            n281 = Increment(x=w609) -> (x+1=w606:i32)
            n282 = In Range and Coerce(upper limit=w606, x=w608, lower limit=w610) -> (coerced(x)=w607:i32)  [unwired: 1 out]
            n283 = Decrement(x=w607) -> (x-1=w605:i32)
            n284 = property on="MCListbox Layout" class="MCListbox (strict)"("Val(Sgnl)"=w605) -> ()  [unwired: 2 in, 2 out]
          }
        }
      }
      event "Layout Browse": Value Change {
        w640 = "_" ("string")
        # "<E7549>"
        # "4070-001-OT02-1001.xls"
        n285 = event-data() -> ()  [unwired: 1 in, 6 out]
        n286 = property on="Layout Details Cluster" class="Clust (strict)"() -> ("Value"=w633:T4)  [unwired: 2 in, 2 out]
        n287 = call "File Dialog"("pattern (all files)"="*.xls") -> ("selected path"=w615:path, "cancelled"=w623:bool, "error out"=w638:errorcluster)  [unwired: 11 in, 1 out]
        "File" <- w638
        "Source path" <- w615
        n288 = Unbundle By Name(w633) -> ("Output Type"=w631:T1, "Layout ID"=w630:T1)
        n289 = property on="Output Set" class="CmbBox (strict)"() -> ("Value"=w632:T1)  [unwired: 2 in, 2 out]
        n290 = global read "Global SRTRS.vi" "Server MasterData\\Layout Folder"() -> (w637:path)
        n291 = local read "[PlantId]"() -> (w641:string)
        n292 = Concatenate Strings(w641, w640, w632, w640, w631, w640, w630, ".xls" ("string")) -> ()  [unwired: 1 out]
        n293 = Path To String(path=w615) -> (string=w626:string)
        n294 = Concatenate Strings(w630, ".xls" ("string")) -> (w628:string)
        n295 = Build Path(base path=w637, name or relative path=w628) -> (appended path=w616:path)
        "Target path" <- w616
        n296 = Path To String(path=w616) -> (string=w625:string)
        n297 = Equal?(x=w616, y=w615) -> (x = y?=w614:bool)
        n298 = case shown="False" w614 {
          tunnel: w638 -> [w648 w649]
          tunnel: w615 -> [w646 _]
          tunnel: w616 -> [w645 _]
          tunnel: [w644 w649] -> w622
          frame False {
            n299 = Copy(8:w648, 9:TRUE ("overwrite (F)"), 10:w645, 11:w646) -> (0:w644:errorcluster)  [unwired: 1 in, 2 out]
          }
          frame True {
            # "Don't Copy if same file\ntreat as no Error"
          }
        }
        n300 = Format Into String(format string="From  \"%s\" to \"%s\". ", w626, w625) -> (resulting string=w624:string)  [unwired: 2 in, 1 out]
        n301 = Path To String(path=w637) -> (string=w642:string)
        n302 = property on="Layout Technical Name" class="Str"(error in=w622, "Val(Sgnl)"=w628) -> (error out=w635:errorcluster)  [unwired: 1 in, 1 out]
        n303 = property on="Layout File Path" class="Str"(error in=w622, "Val(Sgnl)"=w642) -> (error out=w636:errorcluster)  [unwired: 1 in, 1 out]
        n304 = case shown="False" w623 {
          tunnel: w622 -> [w661 _]
          tunnel: w624 -> [w663 _]
          tunnel: [w660 _] -> w621
          tunnel: [w659 _] -> w620
          tunnel: [w658 _] -> w619
          tunnel: [w657 _] -> w617
          tunnel: [w656 _] -> w618
          frame False {
            # "Not Cancelled"
            n305 = case shown="Error" w661 {
              selector: w661 -> [_ w672]
              tunnel: [_ "Layout File Error" ("<.?....> Message Code")] -> w659
              tunnel: [_ w671] -> w664
              tunnel: w663 -> [w665 w670]
              tunnel: [w665 w670] -> w662
              tunnel: [_ "<E 549>" ("<.?....> Message Code")] -> w660
              tunnel: [_ "Error: " ("<.?....> Message Code")] -> w658
              tunnel: [_ TRUE] -> w656
              frame No Error {
                # "File Copy OK."
              }
              frame Error {
                # "{Layout Browse} File Copy Failed."
                n306 = Unbundle By Name(w672) -> ("source"=w671:string)
              }
            }
            n307 = Concatenate Strings(w662, w664) -> (w657:string)
            "File Copy Error" <- w661
          }
          frame True {
            # "Cancelled"
          }
        }
        n308 = Merge Errors(w636, w635) -> (w634:errorcluster)
        n309 = local write "File"(w634) -> ()
        n310 = case shown="True" w618 {
          tunnel: w621 -> [_ w655]
          tunnel: w620 -> [_ w654]
          tunnel: w619 -> [_ w653]
          tunnel: w617 -> [_ w652]
          frame False {
          }
          frame True {
            n311 = call "Msgbox - Message Handler.vi"("Application (Default SRTRS)"="SRTRS", "Short Description (When DB Not Available)"=w654, "Description (When DB Not Available)"=w653, "Post-Description"=w652, "<.?....> Message Code"=w655) -> ("MHandler Error"=w651:errorcluster)  [unwired: 4 in, 2 out]
            n312 = local write "MHandler"(w651) -> ()
          }
        }
      }
      event "SRTRS.MasterData.OutputSet": Value Change {
        w674 = 1  # LayoutFilePath
        # "Applicable only for LayoutId"
        # "Layout Technical Name is updated at Layout Details Cluster Value Change"
        # "Call DB to get values"
        n313 = event-data() -> ("CtlRef"=w710:refnum<vi>)  [unwired: 1 in, 5 out]
        n314 = property class="Str"(reference=w710) -> ("Label.Text"=w708:string, "Value"=w677:string)  [unwired: 1 in, 2 out]
        n315 = Search 1D Array(1D array=w709, element=w708) -> (index of element=w707:i32)  [unwired: 1 in]
        n316 = Index Array(array=w706, index=w707) -> (element=w705:string)
        n317 = Format Into String "[Column Name]"(w705) -> (resulting string=w676:string)  [unwired: 3 in, 1 out]
        "[Column Name] Changed" <- w676
        n318 = case "[Column]" shown="\"LayoutId\"" w676 {
          tunnel: [w713 w718 w726] -> w687
          tunnel: [w714 w716 w722] -> w683
          tunnel: ["USE [<DB>]\n\nSELECT [Description]\nFROM [<Schema>].[<Table>]\n\nWHERE [<A>] = '<B>' AND [PlantID] = '<C>' AND [Inactive] = '0'\n\n" "USE [<DB>]\n\nSELECT [ShortDescription]\nFROM [<Schema>].[<Table>]\n\nWHERE [<A>] = '<B>' AND [Inactive] = '0'\n\n" "USE [<DB>]\n\nSELECT [Description],[LayoutFilePath]\nFROM [<Schema>].[<Table>]\n\nWHERE [<A>] = '<B>' AND [Inactive] = '0'\n\n"] -> w681
          tunnel: w677 -> [_ _ w724]
          frame "OutputSetId", Default {
            n319 = local read "SRTRS.MasterData.OutputSet"() -> (w713:string)
            n320 = control-ref of="Description"() -> (w714:refnum<vi>)
          }
          frame "OutputTypeId" {
            n321 = local read "SRTRS.Config.OutputType"() -> (w718:string)
            n322 = control-ref of="Output Type Description"() -> (w716:refnum<vi>)
          }
          frame "LayoutId" {
            n323 = local read "SRTRS.MasterData.Layout"() -> (w726:string)
            n324 = control-ref of="Layout Description"() -> (w722:refnum<vi>)
            n325 = local read "New Layout Id"() -> (w723:string[])
            n326 = Search 1D Array(1D array=w723, element=w724) -> (index of element=w721:i32)  [unwired: 1 in]
            n327 = case shown="0, Default" w721 {
              tunnel: [T5."Enabled" ("Disabled") T5."Disabled" ("Disabled")] -> w720
              tunnel: [u32 16777215 u32 16777216] -> w719
              frame 0, Default {
              }
              frame -1 {
              }
            }
            n328 = property class="Str"(reference=w722, "DisabledEnum"=w720, "Text.BG Color"=w719) -> ()  [unwired: 1 in, 2 out]
          }
        }
        n329 = call "DB - Split DB.Schema.Table.vi"("DB.Schema.Table"=w687) -> ("DB.Schema.Table"=w698:T15)  [unwired: 10 in]
        n330 = call "DB - Replace DB.Schema.Table.vi"("DB.Schema.Table"=w698, "string in"=w681) -> ("string out"=w691:string)  [unwired: 8 in, 1 out]
        n331 = Search and Replace String(replace all?=TRUE ("replace all? (F)"), input string=w691, search string="<A>", replace string=w676) -> (result string=w690:string)  [unwired: 4 in, 3 out]
        n332 = local read "[PlantId]"() -> (w680:string)
        n333 = Search and Replace String(input string=w690, search string="<B>", replace string=w677) -> (result string=w685:string)  [unwired: 5 in, 3 out]
        n334 = Search and Replace String(input string=w685, search string="<C>", replace string=w680) -> (result string=w679:string)  [unwired: 5 in, 3 out]
        n335 = call-poly <vilib>:"DB Tools Execute Query.vi"("SQL query"=w679, "connection reference"=w686) -> ("error out"=w704:errorcluster, "recordset reference"=w703:T16)  [unwired: 6 in]
        n336 = call-poly <vilib>:"DB Tools Fetch Recordset Data.vi"("error in (no error)"=w704, "recordset reference"=w703) -> ("error out"=w699:errorcluster, "recordset data"=w702:variant[][], "recordset reference out"=w700:T16)  [unwired: 3 in]
        n337 = xnode "Database Variant To Data"("database variant"=w702, "type"=string[][] []) -> ("data"=w696:string[][])  [unwired: 1 in, 1 out]
        n338 = call-poly <vilib>:"DB Tools Free Object.vi"("error in (no error)"=w699, "recordset reference"=w700) -> ("error out"=w692:errorcluster)  [unwired: 8 in, 1 out]
        n339 = Index Array(array=w696, index (row) #1=0 ("disabled index (row)"), index (col) #1=0 ("disabled index (col)"), index (row) #2=0 ("index (row)"), index (col) #2=w674) -> (element #1=w694:string, element #2=w673:string)
        n340 = local write "DB"(w692) -> ()
        n341 = property class="Str"(reference=w683, error in=w692, "Value"=w694) -> (error out=w693:errorcluster)  [unwired: 1 out]
        n342 = case shown="\"LayoutId\"" w676 {
          tunnel: w673 -> [_ w712]
          frame "False", Default {
          }
          frame "LayoutId" {
            n343 = property on="Layout File Path" class="Str"("Value"=w712) -> (error out=w711:errorcluster)  [unwired: 2 in, 1 out]
            n344 = local write "Property Node"(w711) -> ()
          }
        }
        n345 = global write "Global SRTRS.vi" "DB Error"(w692) -> ()
        n346 = local write "Property Node"(w693) -> ()
        n347 = Build Array(w679) -> (w678:string[])
      }
      event "Layout Details Cluster": Value Change {
        w776 = ".xls" ("string")
        w781 = "_" ("string")
        w815 = string[] ["Output Type", "Layout ID", "Layout Description", "Layout Technical Name"]  # 2014-12-05 08:25 ColHdrs[]
        # "4070_005_OT01_111.xls"
        # "Remain T if already T\nUser may have edited current record\nand moved to a new record w/o saving"
        # "Any Changes in Cluster will fire this event. However we cannot detect which Control in the Cluster has changed. \nEach Control in the Cluster must have their own EVENT Change if we want to process that EVENT individually\nSet Save to Enabled if All mandatory Fields filled"
        n348 = event-data() -> ("Time"=→"Layout Details":u32)  [unwired: 1 in, 5 out]
        n349 = property on="MCListbox Layout" class="MCListbox (strict)"() -> ("ItemNames"=w807:string[][], "Value"=w812:i32)  [unwired: 2 in, 2 out]
        n350 = Array Size "Size of ColHdrs[]"(array=w806) -> (size(s)=w805:i32)
        n351 = Array Size(array=w807) -> (size(s)=w813:i32[])
        n352 = Index Array(array=w807, index (row)=w812) -> (element=w804:string[])  [unwired: 1 in]
        n353 = control-ref of="Layout Details Cluster"() -> (w821:refnum<vi>)
        n354 = Array Size(array=w804) -> (size(s)=w808:i32)
        n355 = Index Array(array=w813) -> (element=w810:i32)  [unwired: 1 in]
        n356 = case shown="1, Default" w808 {
          tunnel: w805 -> [w825 _]
          tunnel: w804 -> [_ w827]
          tunnel: [w824 w827] -> w803
          frame 0 {
            # "Create if No Data"
            n357 = Initialize Array("", w825) -> (w824:string[])
          }
          frame 1, Default {
            # "Select Row"
          }
        }
        n358 = property class="Clust (strict)"(reference=w821) -> ("Controls[]"=w820:refnum<vi>[])  [unwired: 1 in, 2 out]
        n359 = local read "Item Number"() -> (w811:i32)
        n360 = Greater?(x=w811, y=w810) -> (0:w796:bool)
        n361 = case shown="True" w796 {
          frame False {
          }
          frame True {
            # "No Row Selected, Must be New Record"
            n362 = local read "New Record in UI not in DB (NA)"() -> (w889:bool)
            n363 = case shown="False" w889 {
              frame False {
                # "New Record NOT Flagged yet."
                n364 = local read "Record Count"() -> (w891:i32)
                n365 = local write "New Record in UI not in DB (NA)"(TRUE ("New Record in UI not in DB")) -> ()
                n366 = Increment(x=w891) -> (x+1=w890:i32)
                n367 = local write "Record Count"(w890) -> ()
                n368 = local write "Current Record"(w890) -> ()
              }
              frame True {
                # "New Record Flagged already\nProbably by NEW Button EVENT"
              }
            }
          }
        }
        n369 = for {
          tunnel: w820 -> [w851] mode=indexing
          tunnel: w806 -> [w850]
          tunnel: [w839] -> w819 mode=indexing
          shift-right: [w845] -> w792
          shift-left: w803 -> [w846]
          tunnel: [w838] -> w816 mode=indexing if=w839
          tunnel: w815 -> [w844]
          w840 = FALSE  # Not Empty
          n370 = property class="Ctl"(reference=w851) -> (reference out=w848:refnum<vi>, "Label.Text"=w838:string, "ClassName"=w847:string)  [unwired: 1 in, 1 out]
          n371 = Search 1D Array(1D array=w850, element=w838) -> (index of element=w849:i32)  [unwired: 1 in]
          n372 = Search 1D Array(1D array=w844, element=w838) -> (index of element=w843:i32)  [unwired: 1 in]
          n373 = Greater Or Equal To 0?(x=w843) -> (x >= 0?=w842:bool)
          n374 = case shown="0, Default" w849 {
            selector: w849 -> [w855 _]
            tunnel: [w860 _] -> w841
            tunnel: w848 -> [w862 _]
            tunnel: w847 -> [w861 _]
            tunnel: w846 -> [w859 w888]
            tunnel: [w858 w888] -> w845
            frame 0, Default {
              # "Cluster Control Found in ColHdrs[]"
              n375 = local read "Col Hdrs[] DB Precision"() -> (w856:string[])
              n376 = local read "Col Hdrs[] DB Data Type"() -> (w857:string[])
              n377 = Index Array(array=w857, index=w855) -> (element=w854:string)
              n378 = Index Array(array=w856, index=w855) -> (element=w853:string)
              n379 = case "Convert to Strings for MCListbox entry" shown="\"ComboBox\", \"String\", Default" w861 {
                tunnel: w862 -> [w868 w877]
                tunnel: [w863 w870] -> w852
                tunnel: w854 -> [_ w873]
                tunnel: w853 -> [_ w872]
                frame "Boolean" {
                  w869 = refnum<vi> refnum  # Boolean
                  n380 = To More Specific Class(target class=w869, reference=w868) -> (specific class reference=w867:refnum<vi>)  [unwired: 1 in, 1 out]
                  n381 = property class="Bool"(reference=w867) -> ("Value"=w866:variant)  [unwired: 1 in, 2 out]
                  n382 = Variant To Data(type=TRUE, Variant=w866) -> (data=w864:bool)  [unwired: 1 in, 1 out]
                  n383 = call "DB - Convert BIT Type.vi"("Boolean"=w864) -> ("BIT (eg Inactive)"=w863:string)  [unwired: 2 in, 2 out]
                }
                frame "ComboBox", "String", Default {
                  w876 = refnum<vi> refnum  # String
                  n384 = To More Specific Class(target class=w876, reference=w877) -> (specific class reference=w875:refnum<vi>)  [unwired: 1 in, 1 out]
                  n385 = property class="Str"(reference=w875) -> (reference out=w871:refnum<vi>, "Value"=w874:string)  [unwired: 1 in, 1 out]
                  n386 = case "CAST TO DB Data Type and Precision" shown="\"int\"" w873 {
                    tunnel: [w880 w883] -> w870
                    tunnel: w872 -> [w878 _]
                    tunnel: w874 -> [w879 w886]
                    frame "nvarchar", Default {
                      n387 = Decimal String To Number(string=w878) -> (number=w881:i32)  [unwired: 2 in, 1 out]
                      n388 = String Subset(string=w879, length (rest)=w881) -> (substring=w880:string)  [unwired: 1 in]
                    }
                    frame "int" {
                      n389 = Decimal String To Number(string=w886) -> (number=w887:i32)  [unwired: 2 in, 1 out]
                      n390 = Empty String/Path?(string/path=w886) -> (empty?=w885:bool)
                      n391 = Number To Decimal String(number=w887) -> (decimal integer string=w884:string)  [unwired: 1 in]
                      n392 = Select(t="", s=w885, f=w884) -> (s? t:f=w883:string)
                    }
                  }
                  n393 = property class="Str"(reference=w871, "Value"=w870) -> ()  [unwired: 1 in, 2 out]
                }
              }
              n394 = Replace Array Subset(array=w859, new element=w852, index=w855) -> (w858:string[])
              n395 = Empty String/Path?(string/path=w852) -> (empty?=w860:bool)
            }
            frame -1 {
            }
          }
          n396 = Select(t=w841, s=w842, f=w840) -> (s? t:f=w839:bool)
        }
        "Empty ColHdrs[]" <- w816
        n397 = property on="Layout Details Cluster" class="Clust (strict)"() -> ("Value"=w780:T4)  [unwired: 2 in, 2 out]
        n398 = Search 1D Array(1D array=w790, element=DB_-_Master_Data_Layout_Enum."b.[LayoutFileName]" ("2014-11-07 13:45\nMaster Data Layout")) -> (index of element=w789:i32)  [unwired: 1 in]
        n399 = Unbundle By Name(w780) -> ("Output Type"=w778:T1, "Layout ID"=w777:T1)
        n400 = property on="Output Set" class="CmbBox (strict)"() -> ("Value"=w779:T1)  [unwired: 2 in, 2 out]
        n401 = local read "[PlantId]"() -> (w782:string)
        n402 = Concatenate Strings(w782, w781, w779, w781, w778, w781, w777, w776) -> ()  [unwired: 1 out]
        n403 = Concatenate Strings(w777, w776) -> (w775:string)
        n404 = global read "Global SRTRS.vi" "Server MasterData\\Layout Folder"() -> (w788:path)
        n405 = Build Path(base path=w788, name or relative path=w775) -> (appended path=w787:path)
        n406 = call <vilib>:"Check if File or Folder Exists.vi"("path"=w787) -> ("file or folder exists?"=w783:bool)  [unwired: 8 in, 2 out]
        n407 = property on="Output Set" class="CmbBox (strict)"() -> ("Value"=w798:T1)  [unwired: 2 in, 2 out]
        n408 = Select(t=w775, s=w783, f="") -> (s? t:f=w784:string)
        n409 = call <vilib>:"Trim Whitespace.vi"("string"=w798) -> ("trimmed string"=w797:string)  [unwired: 1 in]
        n410 = property on="Layout Technical Name" class="Str"("Value"=w784) -> ()  [unwired: 2 in, 2 out]
        n411 = Replace Array Subset(array=w792, new element=w784, index=w789) -> (w785:string[])
        n412 = Replace Array Subset(array=w807, new element=w785, index (row)=w812) -> (w818:string[][])  [unwired: 1 in]
        n413 = case shown="True" w783 {
          tunnel: w818 -> [_ w823]
          frame False {
          }
          frame True {
            # "Only Update if Layout Technical Name OK"
            n414 = property on="MCListbox Layout" class="MCListbox (strict)"("ItemNames"=w823) -> ()  [unwired: 2 in, 2 out]
          }
        }
        n415 = Empty String/Path?(string/path=w797) -> (empty?=w795:bool)
        n416 = Not(x=w795) -> (.not. x?=w793:bool)
        n417 = And(x=w793, y=w796) -> (x .and. y?=w794:bool)
        "Editing Layout Details in New Record" <- w794
        n418 = Or Array Elements(Boolean array=w819) -> (logical OR=w817:bool)
        n419 = Not(x=w817) -> (.not. x?=w809:bool)
        "All Mandatory Fields Filled" <- w809
        n420 = case shown="True" w809 {
          tunnel: [w830 w834] -> w814
          tunnel: w794 -> [_ w837]
          tunnel: [FALSE w833] -> w799
          tunnel: w793 -> [_ w833]
          frame False {
            # "Blank Mandatory Field exsits"
            n421 = Select(t=T5."Disabled and Grayed Out" ("Disabled"), s="Add (Not Save) Enabled depends on \nFilled Mandatory Fields", f=T5."Enabled" ("Disabled")) -> (s? t:f=w830:T5)
          }
          frame True {
            # "All Mandatory Fields Filled"
            n422 = Select(t=T5."Enabled" ("Disabled"), s=w837, f=T5."Disabled and Grayed Out" ("Disabled")) -> (s? t:f=w834:T5)
          }
        }
        n423 = property on="Add" class="Bool"("DisabledEnum"=w814) -> ()  [unwired: 2 in, 2 out]
        n424 = Select(t=T5."Enabled" ("Disabled"), s=w799, f=T5."Disabled and Grayed Out" ("Disabled")) -> (s? t:f=w800:T5)
        n425 = property on="Save" class="Bool"("DisabledEnum"=w800) -> ()  [unwired: 2 in, 2 out]
      }
      event "Add": Value Change {
        # "Set Current Value (Index) to Last Record/Row #"
        n426 = event-data() -> ()  [unwired: 1 in, 6 out]
        n427 = property on="MCListbox Layout" class="MCListbox (strict)"() -> ("ColHdrString"=w913:string[])  [unwired: 2 in, 2 out]
        n428 = local read "Item Number"() -> (w902:i32)
        n429 = Array Size(array=w913) -> (size(s)=w912:i32)
        n430 = property on="Layout Details Cluster" class="Clust (strict)"() -> ("Controls[]"=w898:refnum<vi>[])  [unwired: 2 in, 2 out]
        n431 = Number To Decimal String(number=w902) -> (decimal integer string=w901:string)  [unwired: 1 in]
        n432 = Initialize Array("", w912) -> (w905:string[])
        n433 = control-ref of="Output Set"() -> (w897:refnum<vi>)
        n434 = Replace Array Subset(array=w905, new element=w901, index=0) -> (w903:string[])
        n435 = Build Array (concatenate)(w898, w897) -> (w896:refnum<vi>[])
        n436 = for {
          tunnel: w896 -> [w927] mode=indexing
          tunnel: w913 -> [w925]
          shift-right: [w922] -> w895
          shift-left: w903 -> [w924]
          # "Already CASTED in Cluster Value Change Event"
          # "Convert Controls to Strings for DB\nNo Numeric Controls"
          n437 = property class="Ctl"(reference=w927) -> (reference out=w930:refnum<vi>, "Label.Text"=w926:string, "ClassName"=w928:string, "Value"=w929:variant)  [unwired: 1 in, 1 out]
          n438 = Search 1D Array(1D array=w925, element=w926) -> (index of element=w923:i32)  [unwired: 1 in]
          n439 = case shown="\"ComboBox\", \"String\"" w928 {
            tunnel: w929 -> [w931 w938 _ _]
            tunnel: [w932 w934 "" w940] -> w921
            tunnel: w930 -> [_ _ _ w948]
            frame "ComboBox", "String" {
              n440 = Variant To Data(type="", Variant=w931) -> (data=w932:string)  [unwired: 1 in, 1 out]
            }
            frame "AbsTime" {
              n441 = Variant To Data(type=timestamp(0 s since 1904-01-01), Variant=w938) -> (data=w936:timestamp)  [unwired: 1 in, 1 out]
              n442 = global read "Global SRTRS.vi" "Date Format"() -> (w935:string)
              n443 = Format Date/Time String(time format string (%c)=w935, seconds (now)=w936) -> (date/time string=w934:string)  [unwired: 1 in]
            }
            frame Default {
            }
            frame "Boolean" {
              w947 = refnum<vi> refnum  # Boolean
              n444 = To More Specific Class(target class=w947, reference=w948) -> (specific class reference=w946:refnum<vi>)  [unwired: 1 in, 1 out]
              n445 = property class="Bool"(reference=w946) -> ("Value"=w941:variant)  [unwired: 1 in, 2 out]
              n446 = Variant To Data(type=TRUE, Variant=w941) -> (data=w944:bool)  [unwired: 1 in, 1 out]
              n447 = Select(t="1", s=w944, f="0") -> (s? t:f=w940:string)
            }
          }
          n448 = Replace Array Subset "Create New Record for MCListBox"(array=w924, new element=w921, index=w923) -> (w922:string[])
        }
        n449 = property on="MCListbox Layout" class="MCListbox (strict)"() -> ("ItemNames"=w910:string[][])  [unwired: 2 in, 2 out]
        n450 = Array Size(array=w895) -> (size(s)=w894:i32)
        n451 = Build Array (concatenate)(w910, w895) -> (w908:string[][])
        n452 = Array Size(array=w908) -> (size(s)=w907:i32[])
        n453 = Greater Than 0?(x=w894) -> (x > 0?=w893:bool)
        n454 = Index Array(array=w907) -> (element=w906:i32)  [unwired: 1 in]
        n455 = case shown="True" w893 {
          frame False {
          }
          frame True {
            n456 = property on="Layout ID" class="CmbBox (strict)"() -> ("Value"=w916:T1)  [unwired: 2 in, 2 out]
            n457 = call "Msgbox - Message Handler.vi"("Short Description (When DB Not Available)"="Layout Added", "Description (When DB Not Available)"=" layout added to the output set." ("Short Description (When DB Not Available)"), "Pre-Description"=w916, "<.?....> Message Code"="<I 545>") -> ("MHandler Error"=→"MHandler":errorcluster)  [unwired: 5 in, 2 out]
          }
        }
        n458 = Decrement(x=w906) -> (x-1=w899:i32)
        n459 = property on="MCListbox Layout" class="MCListbox (strict)"("ItemNames"=w908, "Value"=w899) -> (error out=w900:errorcluster)  [unwired: 2 in, 1 out]
        n460 = case shown="0, Default" w899 {
          tunnel: w900 -> [w920 _]
          frame 0, Default {
            n461 = property on="Delete" class="Bool"(error in=w920, "DisabledEnum"=T5."Enabled" ("Disabled")) -> ()  [unwired: 1 in, 2 out]
          }
          frame -1 {
          }
        }
        n462 = property on="Add" class="Bool"("DisabledEnum"=T5."Disabled and Grayed Out" ("Disabled")) -> ()  [unwired: 2 in, 2 out]
      }
      event "Delete": Value Change {
        n463 = event-data() -> ()  [unwired: 1 in, 6 out]
        n464 = property on="Layout ID" class="CmbBox (strict)"() -> ("Value"=w949:T1)  [unwired: 2 in, 2 out]
        n465 = call "Msgbox - Message Handler.vi"("Short Description (When DB Not Available)"="Delete Layout?" ("Description (When DB Not Available)"), "Description (When DB Not Available)"=" layout will be deleted from the output set. Do you want to proceed?", "Pre-Description"=w949, "<.?....> Message Code"="<W 546>" ("Description (When DB Not Available)")) -> ("MHandler Error"=w950:errorcluster, "OK Out"=w951:bool)  [unwired: 5 in, 1 out]
        n466 = local write "MHandler"(w950) -> ()
        n467 = case shown="True" w951 {
          frame False {
          }
          frame True {
            n468 = property on="MCListbox Layout" class="MCListbox (strict)"() -> ("ItemNames"=w969:string[][], "Value"=w966:i32)  [unwired: 2 in, 2 out]
            n469 = Delete From Array(array=w969, index (row)=w966) -> (array with subset deleted=w963:string[][])  [unwired: 2 in, 1 out]
            n470 = local write "Output Set Changed"(TRUE ("Changed")) -> ()
            n471 = Array Size(array=w963) -> (size(s)=w965:i32[])
            n472 = property on="Save" class="Bool"("DisabledEnum"=T5."Enabled" ("Disabled")) -> ()  [unwired: 2 in, 2 out]
            n473 = Decrement(x=w966) -> (x-1=w967:i32)
            n474 = Index Array(array=w965) -> (element=w957:i32)  [unwired: 1 in]
            n475 = for {
              N: w957 -> [_]
              tunnel: [w975] -> w964 mode=indexing
              i -> [w976]
              n476 = Increment(x=w976) -> (x+1=w975:i32)
            }
            n477 = Number To Decimal String(number=w964) -> (decimal integer string=w961:string[])  [unwired: 1 in]
            n478 = Replace Array Subset(array=w963, new element=w961, index (col)=0 ("disabled index (col)")) -> (w959:string[][])  [unwired: 1 in]
            n479 = property on="MCListbox Layout" class="MCListbox (strict)"("ItemNames"=w959, "Val(Sgnl)"=w967) -> ()  [unwired: 2 in, 2 out]
            n480 = Array Size(array=w959) -> (size(s)=w958:i32[])
            n481 = Index Array(array=w958) -> (element=w956:i32)  [unwired: 1 in]
            n482 = Greater?(x=w957, y=w956) -> (0:w955:bool)
            n483 = case shown="True" w955 {
              frame False {
              }
              frame True {
                n484 = property on="Layout ID" class="CmbBox (strict)"() -> ("Value"=w970:T1)  [unwired: 2 in, 2 out]
                n485 = call "Msgbox - Message Handler.vi"("Short Description (When DB Not Available)"="Layout Deleted" ("Description (When DB Not Available)"), "Description (When DB Not Available)"=" layout deleted.", "Pre-Description"=w970, "<.?....> Message Code"="<I 547>" ("Description (When DB Not Available)")) -> ("MHandler Error"=w971:errorcluster)  [unwired: 5 in, 2 out]
                n486 = local write "MHandler"(w971) -> ()
              }
            }
          }
        }
      }
      event "------------------------------------        MCListBox EVENTS     ------------------------------------   3": Value Change {
        n487 = event-data() -> ()  [unwired: 1 in, 6 out]
      }
      event "MCListbox Layout": Value Change {
        # "USER Clicks on MCListbox\nDisable Save, Updates Details Header Cluster"
        n488 = event-data() -> ("Time"=→"MCListBox":u32, "NewVal"=w982:i32)  [unwired: 1 in, 4 out]
        "NewVal" <- w982
        n489 = disable-structure shown="Disabled" {
          frame Disabled {
            n490 = property on="Save" class="Bool"("DisabledEnum"=T5."Disabled and Grayed Out" ("Disabled")) -> ()  [unwired: 2 in, 2 out]
          }
          frame Enabled {
          }
        }
        n491 = property on="Layout Description" class="Str"("DisabledEnum"=T5."Disabled" ("Disabled"), "Text.BG Color"=u32 16777216) -> ()  [unwired: 2 in, 2 out]
        n492 = flat-sequence {
          tunnel: w982 -> [w988]
          frame #0 {
            # "MClistBox Value Change EVENT\nThis Sequence Controls the ItemNo to show the Next Available Blank Record of the MCListBox\nThe other Suquence will be in the ItemNo Value Change EVENT which sets the MCListBox Value"
            n493 = property on="MCListbox Layout" class="MCListbox (strict)"() -> ("ItemNames"=w984:string[][])  [unwired: 2 in, 2 out]
            n494 = Array Size(array=w984) -> (size(s)=w989:i32[])
            n495 = Index Array(array=w989) -> (element=w987:i32)  [unwired: 1 in]
            n496 = case shown="0, Default" w988 {
              selector: w988 -> [w991 _]
              tunnel: [w996 w998] -> w986
              tunnel: w987 -> [w995 w999]
              tunnel: [w993 T5."Disabled and Grayed Out" ("Disabled")] -> w985
              frame 0, Default {
                # "Disable Delete if new Record"
                # "0 to LastValue+1"
                n497 = Increment(x=w991) -> (x+1=w996:i32)
                n498 = Greater?(x=w996, y=w995) -> (0:w994:bool)
                n499 = Select(t=T5."Disabled and Grayed Out" ("Disabled"), s=w994, f=T5."Enabled" ("Disabled")) -> (s? t:f=w993:T5)
              }
              frame -1 {
                # "Nothing Selected\nGOTO next Record/Row"
                n500 = Increment(x=w999) -> (x+1=w998:i32)
              }
            }
            n501 = local write "Item Number"(w986) -> ()
            n502 = local write "Current Record"(w986) -> ()
            n503 = property on="Delete" class="Bool"("DisabledEnum"=w985) -> ()  [unwired: 2 in, 2 out]
          }
        }
        n504 = disable-structure shown="Disabled" {
          frame Disabled {
            n505 = local read "New Record in UI not in DB (NA)"() -> (w1000:bool)
            n506 = case shown="True" w1000 {
              frame False {
                # "Current Record Count is correct"
              }
              frame True {
                # "Current Record Count must -1 since New Record\nno longer available and NOT in DB"
                n507 = local read "Record Count"() -> (w1003:i32)
                n508 = local write "New Record in UI not in DB (NA)"(FALSE ("New Record in UI not in DB")) -> ()
                n509 = Decrement(x=w1003) -> (x-1=w1002:i32)
                n510 = local write "Record Count"(w1002) -> ()
              }
            }
          }
          frame Enabled {
          }
        }
        n511 = property on="Layout Details Cluster" class="Clust (strict)"() -> (error out=w980:errorcluster, "Controls[]"=w981:refnum<vi>[])  [unwired: 2 in, 1 out]
        n512 = for {
          tunnel: w981 -> [w1018] mode=indexing
          tunnel: w982 -> [w1007]
          tunnel: [w1011] -> w979
          tunnel: w980 -> [w1009]
          n513 = property on="MCListbox Layout" class="MCListbox (strict)"() -> ("ColHdrString"=w1017:string[], "ItemNames"=w1008:string[][])  [unwired: 2 in, 2 out]
          n514 = Index Array(array=w1008, index (row)=w1007, index (col)=0 ("disabled index (col)")) -> (element=w1005:string)
          n515 = property on="Search User ID" class="CmbBox (strict)"("Value"=w1005) -> ()  [unwired: 2 in, 2 out]
          n516 = property class="Ctl"(reference=w1018, error in=w1009) -> (reference out=w1012:refnum<vi>, error out=w1010:errorcluster, "Label.Text"=w1016:string)
          n517 = local read "Col Hdrs[] DB Data Type"() -> (w1013:string[])
          n518 = Search 1D Array(1D array=w1017, element=w1016) -> (index of element=w1014:i32)  [unwired: 1 in]
          n519 = Greater Or Equal To 0?(x=w1014) -> (x >= 0?=w1015:bool)
          n520 = case shown="True" w1015 {
            tunnel: w1008 -> [_ w1030]
            tunnel: w1007 -> [_ w1029]
            tunnel: w1014 -> [_ w1027]
            tunnel: w1013 -> [_ w1028]
            tunnel: w1012 -> [_ w1025]
            tunnel: [w1019 w1022] -> w1011
            tunnel: w1010 -> [w1019 w1021]
            frame False {
            }
            frame True {
              # "Not used"
              n521 = Index Array(array=w1030, index (row)=w1029, index (col)=w1027) -> (element=w1026:string)
              n522 = Index Array(array=w1028, index=w1027) -> ()  [unwired: 1 out]
              n523 = property class="Ctl"(reference=w1025, error in=w1021) -> (reference out=w1023:refnum<vi>, error out=w1020:errorcluster, "ClassName"=w1024:string)
              n524 = case shown="\"Boolean\"" w1024 {
                tunnel: w1026 -> [w1033 w1045 w1051]
                tunnel: w1023 -> [w1034 w1039 w1055]
                tunnel: [w1032 w1036 w1052] -> w1022
                tunnel: w1020 -> [w1031 w1035 _]
                frame "False", Default {
                  n525 = property class="Ctl"(reference=w1034, error in=w1031, "Value"=w1033) -> (error out=w1032:errorcluster)  [unwired: 1 out]
                }
                frame "Boolean" {
                  w1040 = refnum<vi> refnum  # Boolean
                  n526 = Equal?(x="1", y=w1045) -> (x = y?=w1043:bool)
                  n527 = Select(t=TRUE, s=w1043, f=FALSE) -> (s? t:f=w1037:bool)
                  n528 = To More Specific Class(target class=w1040, reference=w1039) -> (specific class reference=w1038:refnum<vi>)  [unwired: 1 in, 1 out]
                  n529 = property class="Bool"(reference=w1038, error in=w1035, "Value"=w1037) -> (error out=w1036:errorcluster)  [unwired: 1 out]
                }
                frame "AbsTime" {
                  w1054 = refnum<vi> refnum  # AbsTime
                  n530 = call "String - Convert Str (YYYY-mm-dd HHcMMcSS) to TimeStamp.vi"("YYYY-mm-dd HH:MM:SS (String)"=w1051) -> ("time stamp"=w1046:timestamp)  [unwired: 9 in, 1 out]
                  n531 = To More Specific Class(target class=w1054, reference=w1055) -> (specific class reference=w1053:refnum<vi>)  [unwired: 1 in, 1 out]
                  n532 = Greater?(x=w1046, y=timestamp(31593600 s since 1904-01-01)) -> (0:w1049:bool)
                  n533 = Select(t=w1046, s=w1049, f=timestamp(0 s since 1904-01-01) ("time stamp")) -> (s? t:f=w1048:timestamp)
                  n534 = property class="AbsTime"(reference=w1053, "Value"=w1048) -> (error out=w1052:errorcluster)  [unwired: 1 in, 1 out]
                }
              }
            }
          }
        }
        n535 = local write "Property Node"(w979) -> ()
      }
      event "------------------------------------------        Unused EVENTS     ----------------------------------------": Value Change {
        # "EVENTS Not used in this VI"
        n536 = event-data() -> ()  [unwired: 1 in, 6 out]
      }
      event "Next Button", "Previous Button", "Last Button", "First Button", "Include Inactive": Value Change {
        # "NOT used in DB UI - Admin User"
        n537 = event-data() -> ("CtlRef"=w1056:refnum<vi>)  [unwired: 1 in, 5 out]
        n538 = disable-structure shown="Disabled" {
          disable-tunnel: [w1060 _] -> _
          disable-tunnel: w1058 -> [w1066 _]
          disable-tunnel: w1057 -> [w1065 _]
          disable-tunnel: w1056 -> [w1059 _]
          frame Disabled {
            n539 = control-ref of="Include Inactive"() -> (w1061:refnum<vi>)
            n540 = local read "New Record in UI not in DB (NA)"() -> (w1063:bool)
            n541 = Equal?(x=w1059, y=w1061) -> (x = y?=w1060:bool)
            n542 = case shown="True" w1063 {
              tunnel: [_ errorcluster {"status"=FALSE, "code"=0, "source"=""} ("error constant")] -> w1062
              frame False {
              }
              frame True {
                n543 = local read "Record Count"() -> (w1078:i32)
                n544 = local write "New Record in UI not in DB (NA)"(FALSE ("New Record in UI not in DB")) -> ()
                n545 = Decrement(x=w1078) -> (x-1=w1077:i32)
                n546 = local write "Record Count"(w1077) -> ()
              }
            }
            n547 = Build Array("First Button", "Previous Button", "Next Button", "Last Button", w1060) -> (w1071:bool[])
            n548 = Search 1D Array(1D array=w1071, element=TRUE) -> (index of element=w1064:i32)  [unwired: 1 in]
            n549 = property on="Current Record" class="DigNum (strict)"() -> ("Value"=w1075:i32)  [unwired: 2 in, 2 out]
            n550 = case shown="4" w1064 {
              tunnel: w1075 -> [_ w1083 w1085 _ w1087]
              tunnel: [1 w1082 w1084 w1086 w1087] -> w1074
              tunnel: w1066 -> [_ _ _ _ _]
              tunnel: w1065 -> [_ _ _ _ _]
              tunnel: w1062 -> [_ _ _ _ _]
              frame 0, Default {
                # "1st Record"
              }
              frame 1 {
                # "Previous"
                n551 = Decrement(x=w1083) -> (x-1=w1082:i32)
              }
              frame 2 {
                # "Next"
                n552 = Increment(x=w1085) -> (x+1=w1084:i32)
              }
              frame 3 {
                # "Last Record"
                n553 = local read "Record Count"() -> (w1086:i32)
              }
              frame 4 {
                # "Refresh the entireTable because we need to update # of Records also"
                # "Include Invalid"
                n554 = disable-structure shown="Disabled" {
                  frame Disabled {
                    n555 = property on="Property Node" class="CmbBox (strict)"() -> (reference out=w1088:refnum<vi>, "Value"=w1089:T1)  [unwired: 2 in, 1 out]
                    n556 = property on="Property Node" class="CmbBox (strict)"(reference=w1088, "Val(Sgnl)"=w1089) -> ()  [unwired: 1 in, 2 out]
                  }
                  frame Enabled {
                  }
                }
              }
            }
            n557 = case shown="0, Default" w1064 {
              tunnel: w1074 -> [w1080 _]
              frame 0, Default {
                # "Update MCListBox"
                n558 = property on="Current Record" class="DigNum (strict)"("Val(Sgnl)"=w1080) -> ()  [unwired: 2 in, 2 out]
              }
              frame 4 {
                # "Event already FIRED in Select Table"
              }
            }
            n559 = local write "Output Set Changed"(FALSE ("Changed")) -> ()
          }
          frame Enabled {
          }
        }
      }
      event Value Change {
        # "Show Searched Row as Top Row"
        # "Leave 5 Rows on top"
        n560 = event-data() -> ("NewVal"=w1097:T1)  [unwired: 1 in, 5 out]
        n561 = property class="MCListbox (strict)"(reference=w1101) -> ("ItemNames"=w1100:string[][])  [unwired: 1 in, 2 out]
        n562 = Index Array(array=w1100, index (col)=0 ("disabled index (col)")) -> (element=w1098:string[])  [unwired: 1 in]
        n563 = Search 1D Array(1D array=w1098, element=w1097) -> (index of element=w1090:i32)  [unwired: 1 in]
        n564 = Subtract(x=w1090, y=5) -> (x-y=w1092:i32)
        n565 = Greater Or Equal To 0?(x=w1092) -> (x >= 0?=w1093:bool)
        n566 = Select(t=w1092, s=w1093, f=0) -> ()  [unwired: 1 out]
        n567 = Bundle("index of element"=w1090, 0) -> (w1094:cluster{"index of element":i32, i32})  [unwired: 1 in]
        n568 = property on="MCListbox Layout" class="MCListbox (strict)"("Val(Sgnl)"=w1090, "TopLeft"=w1094) -> ()  [unwired: 2 in, 2 out]
      }
      event "Current Record": Value Change {
        n569 = event-data() -> ()  [unwired: 1 in, 6 out]
        n570 = local read "Record Count"() -> (w1105:i32)
        n571 = In Range and Coerce(upper limit=w1105, x="Current Record", lower limit=1) -> (coerced(x)=w1106:i32, In Range?=w1102:bool)
        n572 = control-ref of="Current Record"() -> (w1104:refnum<vi>)
        n573 = case shown="False" w1102 {
          tunnel: w1110 -> [w1113 w1114]
          tunnel: w1106 -> [w1111 w1115]
          tunnel: [w1113 w1114] -> w1109
          tunnel: w1108 -> [_ _]
          tunnel: "Current Record" -> [_ _]
          tunnel: w1104 -> [w1112 w1116]
          frame False {
            # "To fire an event again so\nthat the calling VIs gets notified\n\nIt may mean that the same record will \nbe fetched again"
            # "Coerce back to Record #"
            n574 = property class="DigNum (strict)"(reference=w1112, "Val(Sgnl)"=w1111) -> ()  [unwired: 1 in, 2 out]
          }
          frame True {
            # "Valid Record#"
            n575 = property class="DigNum (strict)"(reference=w1116, "Value"=w1115) -> ()  [unwired: 1 in, 2 out]
          }
        }
      }
    }
    "Statemachine" <- w103
    "SQL" <- w92
  }
  n576 = disable-structure shown="Disabled" {
    frame Disabled {
      w1118 = "%Y-%m-%d %H:%M:%S"  # SQL Server datetime
      n577 = Get Date/Time In Seconds() -> (seconds since 1Jan1904=w1119:timestamp)
      n578 = Format Date/Time String(time format string (%c)=w1118, seconds (now)=w1119) -> (date/time string=w1117:string)  [unwired: 1 in]
      "datetime string" <- w1117
      n579 = Concatenate Strings("INSERT INTO " ("string"), "(TStamp)" ("string"), " values " ("string"), "('" ("string"), w1117, "')" ("string")) -> ()  [unwired: 1 in, 1 out]
    }
    frame Enabled {
    }
  }
  n580 = call <vilib>:"DB Tools Close Connection.vi"("error in (no error)"=w14, "connection reference"=w15) -> ("error out"=→"Close":errorcluster)  [unwired: 5 in]
